vi "Receive TCP Message.vi"(3 "Error In":errorcluster, 4 "TCP Network Connection Refnum":refnum<k5>, 5 "Supervisor In":refnum<class "Supervisor.lvclass">) -> (0 "Error Out":errorcluster, 1 "TCP Network Connection Refnum Out":refnum<k5>, 2 "Supervisor Out":refnum<class "Supervisor.lvclass">)   [LabVIEW 2014, in "Supervisor.lvclass"]
uses:
  Supervisor.lvclass
  Supervisor.lvclass/Supervisor.ctl
panel:
  out "Numeric":i32
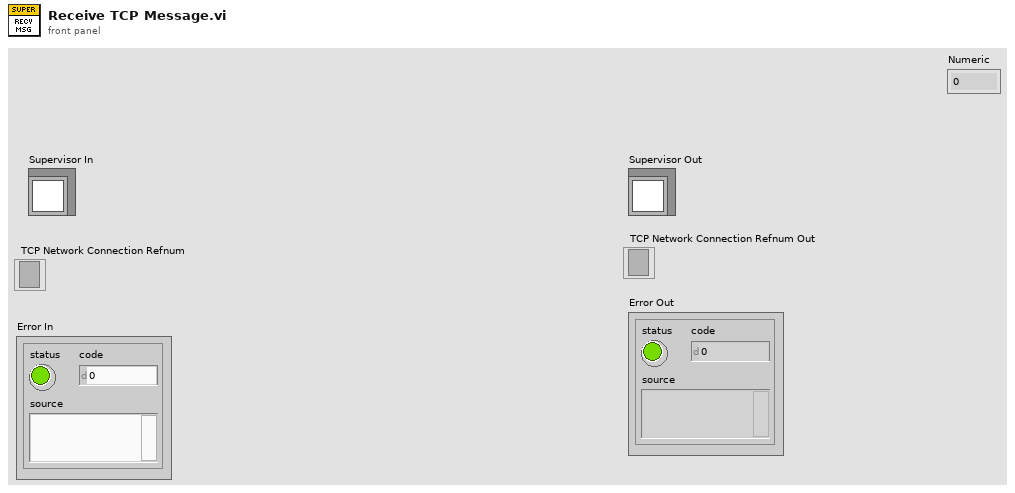
[diagram p1: front panel]
types:
  T1 = cluster{"javp":dbl[], " javr":dbl[], "Break":bool, "arrived":bool, "arrived yaw":bool}
  T2 = typedef "nicrio_cRIO-9871_BaudRateEnum.ctl" = enum16{"75 bps", "110 bps", "134 bps", "150 bps", "300 bps", "600 bps", "1200 bps", "1800 bps", "2400 bps", "4800 bps", "7200 bps", "9600 bps", "14.4 kbps", "19.2 kbps", "28.8 kbps", "38.4 kbps", "57.6 kbps", "115.2 kbps", "230.4 kbps", "460.8 kbps", "921.6 kbps"}
  T3 = typedef "nicrio_cRIO-9871_DataBitsEnum.ctl" = enum8{"5", "6", "7", "8"}
  T4 = typedef "nicrio_cRIO-9871_ParityEnum.ctl" = enum8{"None", "Odd", "Even", "Mark", "Space"}
  T5 = typedef "nicrio_cRIO-9871_StopBitsEnum.ctl" = enum8{"1", "1.5", "2"}
  T6 = typedef "nicrio_cRIO-9871_FlowControlEnum.ctl" = enum8{"None", "Software (XON / XOFF)", "Hardware (RTS / CTS)"}
  T7 = cluster{"Baud Rate":T2, "Data Bits":T3, "Parity":T4, "Stop Bits":T5, "Flow Control":T6}[]
  T8 = cluster{"Baud Rate":T2, "Data Bits":T3, "Parity":T4, "Stop Bits":T5, "Flow Control":T6}
  T9 = typedef "NI_Matrix.lvlib/RealMatrix.ctl" = dbl[][]
  T10 = cluster{"Performance Behavior":cluster{"% Velocity max lin to exp":dbl, "% Velocity zero lin to exp":dbl, "% Total dist at max velocity":dbl, "Max angular velocity":dbl, "Time to max linear velocity":dbl, "Min dist at max velocity":dbl, "Max linear velocity":dbl, "Time to max angular velocity":dbl}, "Table of WP":dbl[][], "Tracking Options":cluster{"Superior Bound":dbl, "Inferior Bound":dbl, "Duration No operation period between motions":dbl, "Tolerance of initial angle":dbl, "Distance to activation waiting function":dbl, "Distance to deactivation waiting function":dbl, "(2) Fixed Heading":dbl, "(3) PoI N":dbl, "(3) PoI E":dbl}, "Start":bool, "Use Position":bool, "Heading Mode":u16, "Pause":bool, "Abort":bool}
  T11 = cluster{"R":T9, "Q":T9, "Update R":bool, "Update Q":bool, "Name":string}
  T12 = cluster{"KP":T9, "KD":T9, "KI":T9, "KA":T9, "Update KP":bool, "Update KD":bool, "Update KI":bool, "Update KA":bool, "Name":string}
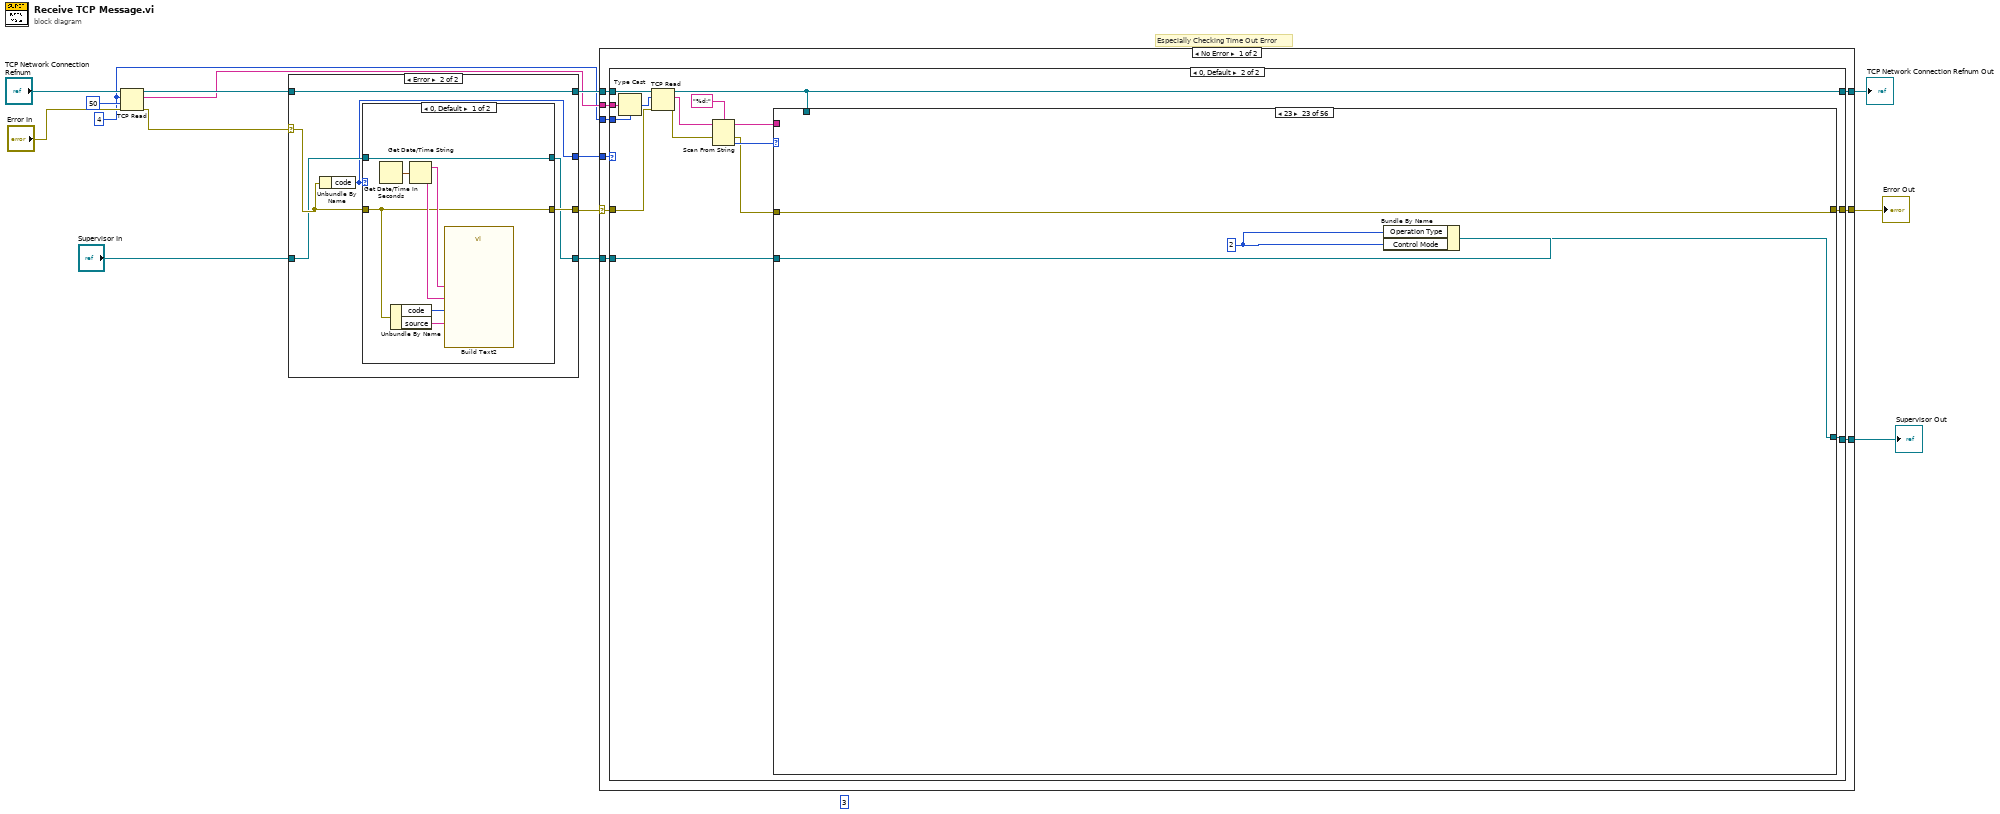
[diagram p0: block diagram]
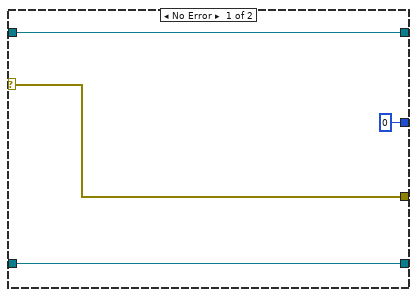
[diagram p2: hidden frame]
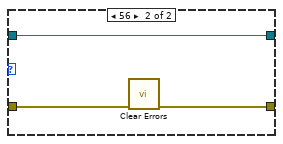
[diagram p3: hidden frame]
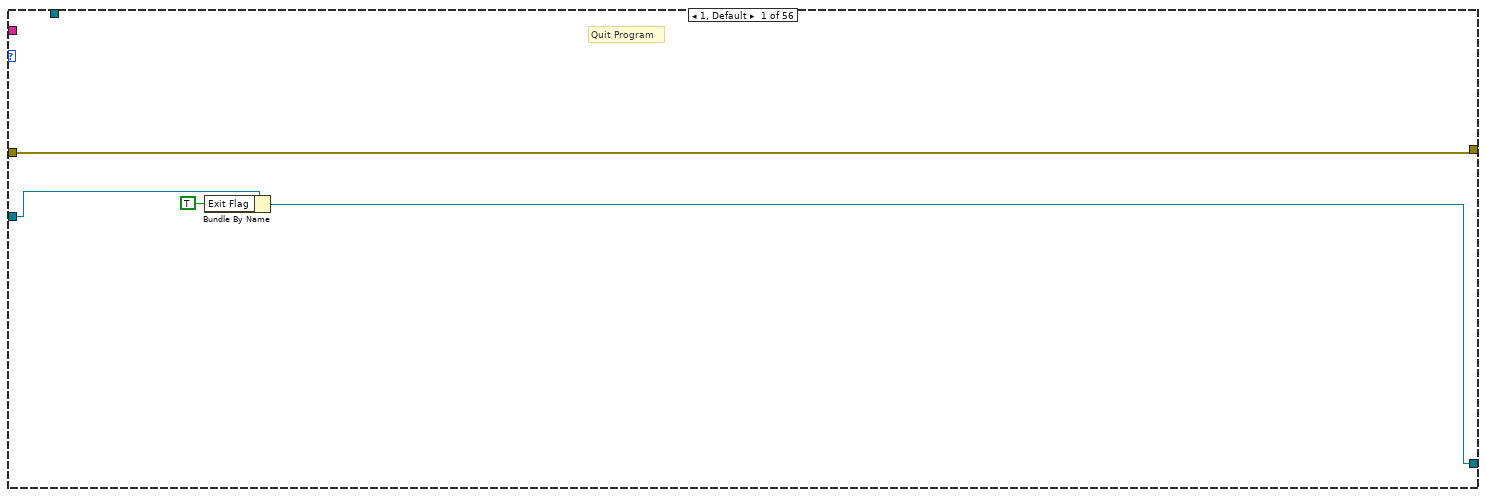
[diagram p5: hidden frame]
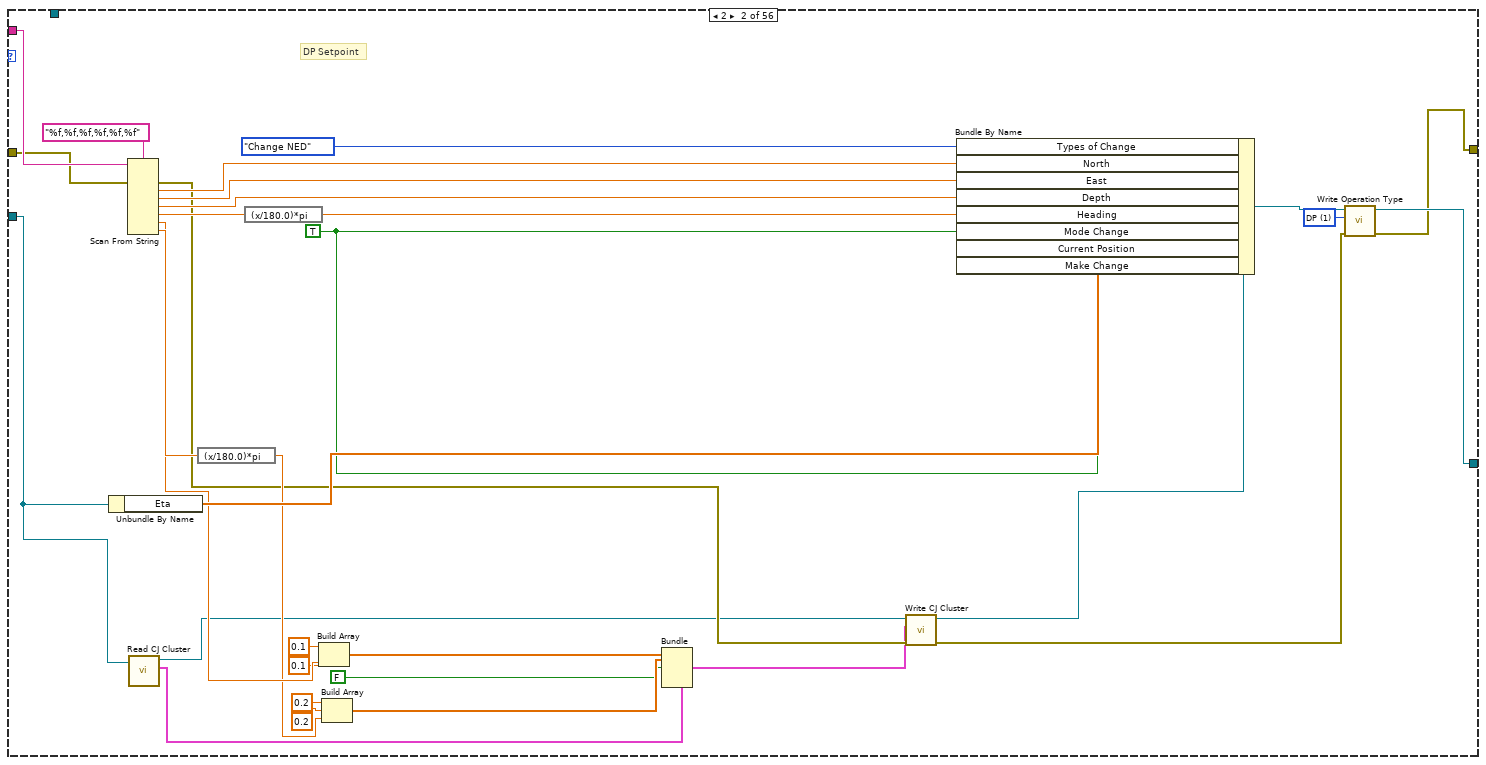
[diagram p6: hidden frame]
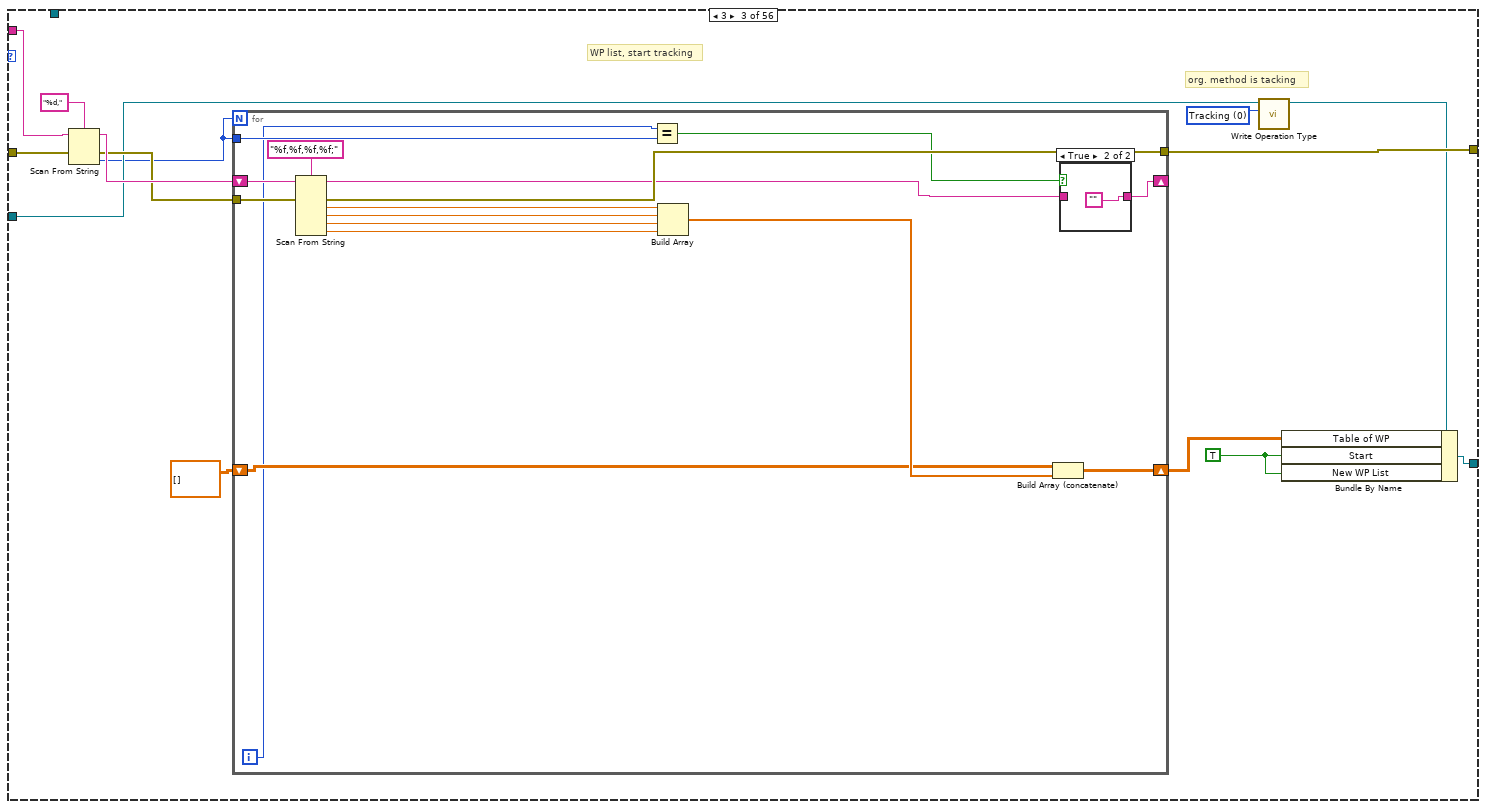
[diagram p7: hidden frame]
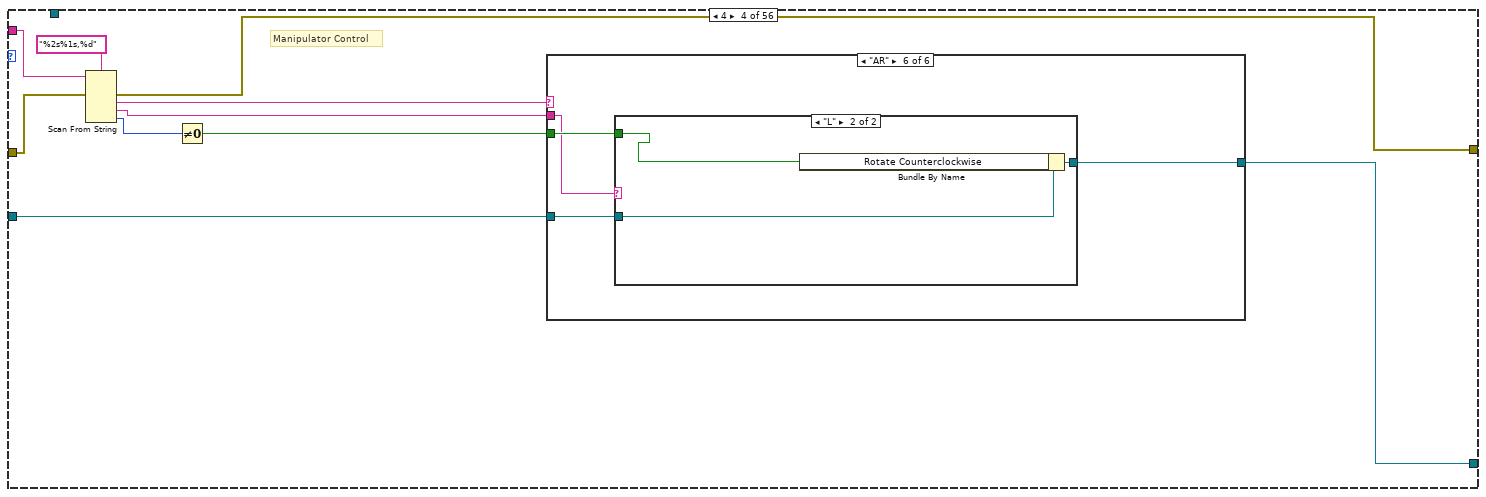
[diagram p9: hidden frame]
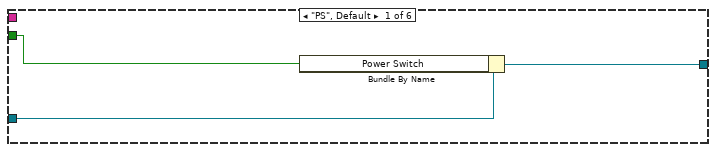
[diagram p10: hidden frame]
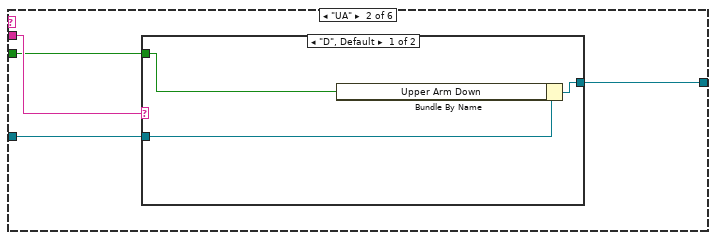
[diagram p11: hidden frame]
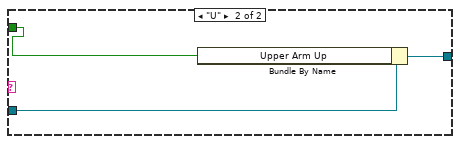
[diagram p12: hidden frame]
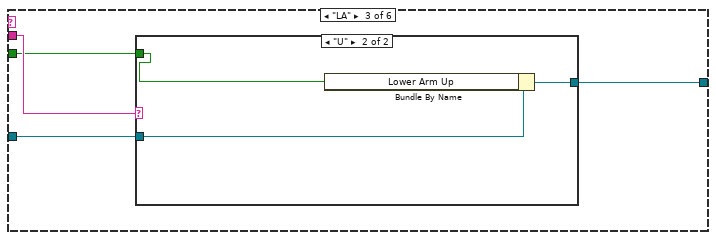
[diagram p13: hidden frame]
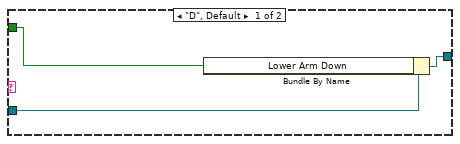
[diagram p14: hidden frame]
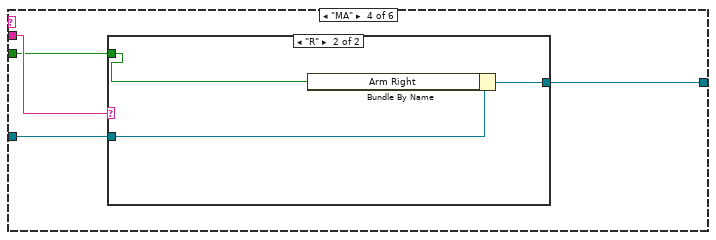
[diagram p15: hidden frame]
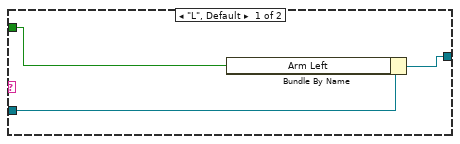
[diagram p16: hidden frame]
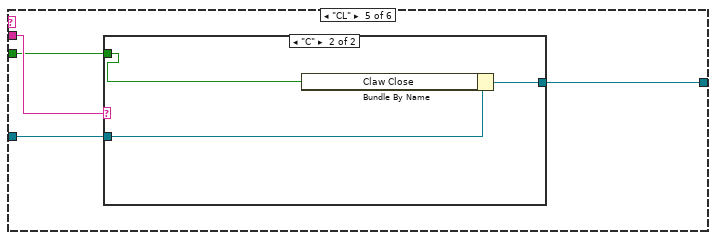
[diagram p17: hidden frame]
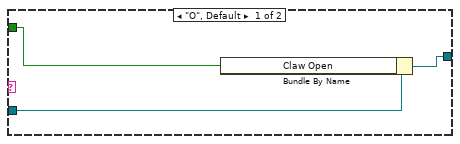
[diagram p18: hidden frame]
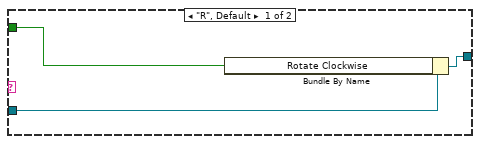
[diagram p19: hidden frame]
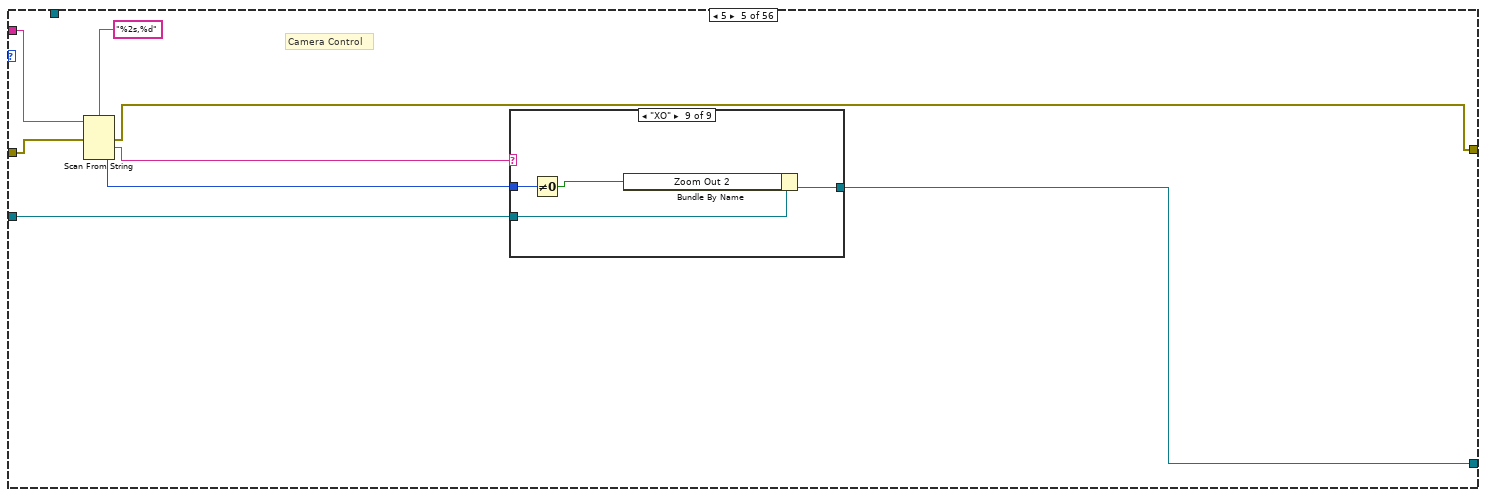
[diagram p20: hidden frame]
diagram:
  (unwired) 3
  w2 = 4
  # "Especially Checking Time Out Error"
  n1 = TCP Read(connection ID="TCP Network Connection Refnum", bytes to read=w2, error in (no error)="Error In", 9:50 ("timeout ms (25000)")) -> (connection ID out=w6:refnum<k5>, data out=w4:string, error out=w5:errorcluster)  [unwired: 1 in]
  n2 = case shown="Error" w5 {
    selector: w5 -> [w17 w24]
    tunnel: w6 -> [w19 w25]
    tunnel: [w19 w25] -> w9
    tunnel: [w18 w21] -> w8
    tunnel: [w17 w23] -> w3
    tunnel: "Supervisor In" -> [w18 w22]
    tunnel: [0 ("code") w20] -> w1
    frame No Error {
    }
    frame Error {
      n3 = Unbundle By Name(w24) -> ("code"=w20:i32)
      n4 = case shown="0, Default" w20 {
        tunnel: w24 -> [w29 w35]
        tunnel: [w29 w34] -> w23
        tunnel: w22 -> [w26 w33]
        tunnel: [w26 w33] -> w21
        frame 0, Default {
          n5 = Get Date/Time In Seconds() -> (seconds since 1Jan1904=w32:timestamp)
          n6 = Unbundle By Name(w29) -> ("code"=w28:i32, "source"=w27:string)
          n7 = Get Date/Time String(seconds (now)=w32) -> (date string=w31:string, time string=w30:string)  [unwired: 2 in]
          n8 = call "Build Text2"("Msg"=w27, "Date"=w31, "Time"=w30, "Code"=w28) -> ()  [unwired: 10 in, 2 out]
        }
        frame 56 {
          n9 = call <vilib>:"Clear Errors.vi"("error in (no error)"=w35) -> ("error out"=w34:errorcluster)  [unwired: 5 in, 1 out]
        }
      }
    }
  }
  n10 = case shown="No Error" w3 {
    selector: w3 -> [w38 w1206]
    tunnel: w9 -> [w44 w1210]
    tunnel: w4 -> [w43 _]
    tunnel: w2 -> [w42 _]
    tunnel: [w41 w1210] -> w14
    tunnel: [w40 w1207] -> w13
    tunnel: [w39 w1205] -> w11
    tunnel: w8 -> [w37 w1208]
    tunnel: w1 -> [w36 _]
    frame No Error {
      n11 = case shown="0, Default" w36 {
        tunnel: w44 -> [w47 w62]
        tunnel: w43 -> [_ w61]
        tunnel: w42 -> [_ w60]
        tunnel: [w47 w48] -> w41
        tunnel: [w45 w54] -> w40
        tunnel: [w46 w51] -> w39
        tunnel: w38 -> [w46 w50]
        tunnel: w37 -> [w45 w49]
        frame 56 {
        }
        frame 0, Default {
          n12 = Type Cast(type=w60, x=w61) -> (*(type *) &x=w59:i32)
          n13 = TCP Read(connection ID=w62, bytes to read=w59, error in (no error)=w50) -> (connection ID out=w48:refnum<k5>, data out=w58:string, error out=w53:errorcluster)  [unwired: 2 in]
          n14 = Scan From String(format string="%d:", input string=w58, error in=w53) -> (remaining string=w55:string, error out=w52:errorcluster, output 1=w56:i32)  [unwired: 2 in, 1 out]
          n15 = case shown="23" w56 {
            selector: w56 -> [_ _ _ _ _ _ w297 _ _ _ _ _ _ _ _ _ _ _ _ _ _ _ _ _ _ _ _ _ _ _ _ _ _ _ _ _ _ _ _ _ _ _ _ _ _ _ _ _ _ _ _ _ _ _ _ _]
            tunnel: w55 -> [_ w97 w111 w140 w199 w244 _ w307 w366 w420 w446 w466 w473 w483 w495 _ _ _ w529 w756 w764 w769 _ w782 w790 w795 w805 w809 w817 w827 w835 w843 w851 w859 w872 w911 w919 _ w943 w967 w976 w997 w1008 w1016 w1033 w1039 w1048 w1056 _ _ w1157 w1164 w1176 w1186 w1191 w1202]
            tunnel: w49 -> [w66 w68 w103 w134 w201 w240 w296 w302 w364 w418 w447 w463 w475 w480 w491 w509 w512 w516 w528 w753 w761 w768 w776 w779 w792 w797 w804 w813 w821 w829 w837 w845 w853 w861 w867 w908 w914 w923 w946 w968 w974 w985 w1007 w1015 w1031 w1037 w1043 w1054 w1086 w1122 w1161 w1169 w1174 w1183 w1190 w1199]
            tunnel: [w64 w88 w107 w133 w196 w239 w296 w301 w363 w416 w439 w459 w469 w476 w487 w507 w511 w515 w527 w751 w759 w766 w774 w777 w791 w796 w803 w812 w820 w828 w836 w841 w852 w860 w865 w906 w912 w923 w940 w966 w973 w982 w1000 w1013 w1024 w1035 w1045 w1053 w1086 w1122 w1160 w1163 w1173 w1184 w1189 w1197] -> w54
            tunnel: w52 -> [w63 w90 w106 w132 w195 w238 w295 w300 w365 w415 w444 w461 w474 w484 w492 w506 w513 w517 w526 w750 w758 w770 w773 w781 w786 w794 w802 w811 w819 w826 w834 w844 w850 w858 w871 w905 w917 w922 w947 w969 w975 w996 w1009 w1017 w1032 w1038 w1047 w1052 w1088 w1149 w1156 w1168 w1177 w1185 w1192 w1203]
            tunnel: [w63 w74 w104 w131 w194 w237 w295 w298 w394 w414 w443 w458 w467 w479 w490 w506 w513 w517 w524 w749 w757 w765 w773 w780 w785 w793 w801 w810 w818 w825 w833 w842 w849 w857 w870 w904 w915 w921 w939 w965 w972 w981 w999 w1014 w1025 w1036 w1046 w1050 w1087 w1148 w1162 w1166 w1171 w1180 w1193 w1198] -> w51
            tunnel: w48 -> [_ _ _ _ _ _ _ _ _ _ _ _ _ _ _ _ _ _ _ _ _ _ _ _ _ _ _ _ _ _ _ _ _ _ _ _ _ w920 _ _ _ _ _ _ _ _ _ _ w1089 w1150 _ _ _ _ _ _]
            frame 1, Default {
              # "Quit Program"
              n16 = Bundle By Name(cluster=w66, "Exit Flag"=TRUE) -> (w64:refnum<class "Supervisor.lvclass">)
            }
            frame 2 {
              w87 = u16 1 items=["Tracking", "DP", "Joystick"] ("Operation Type")
              w91 = TRUE ("Guidance Cluster.Update Reference.Mode Change")
              # "DP Setpoint"
              n17 = Unbundle By Name(w68) -> ("Eta"=w92:dbl[])
              n18 = Scan From String(format string="%f,%f,%f,%f,%f,%f", input string=w97, error in=w90) -> (error out=w75:errorcluster, output 1=w96:dbl, output 2=w95:dbl, output 3=w94:dbl, output 4=w85:dbl, output 5=w83:dbl, output 6=w84:dbl)  [unwired: 7 in, 2 out]
              n19 = call-dynamic "Read CJ Cluster.vi"("Supervisor in"=w68) -> ("CJ Cluster"=w71:T1, "Supervisor out"=w67:refnum<class "Supervisor.lvclass">)  [unwired: 8 in, 1 out]
              n20 = expression code="(x/180.0)*pi" ("degrees to radians")(w84) -> (w78:dbl)
              n21 = expression code="(x/180.0)*pi" ("degrees to radians")(w85) -> (w86:dbl)
              n22 = Build Array(0.1 ("element"), 0.1 ("element"), w83) -> (w77:dbl[])
              n23 = Build Array(0.2 ("element"), 0.2 ("element"), w78) -> (w73:dbl[])
              n24 = Bundle(cluster=w71, "javp"=w77, "javr"=w73, "Break"=FALSE ("Guidance Cluster.Update Reference.Mode Change")) -> (w70:T1)  [unwired: 2 in]
              n25 = call-dynamic "Write CJ Cluster.vi"("error in (no error)"=w75, "CJ Cluster"=w70, "Supervisor in"=w67) -> ("error out"=w76:errorcluster, "Supervisor out"=w72:refnum<class "Supervisor.lvclass">)  [unwired: 7 in]
              n26 = Bundle By Name(cluster=w72, "Types of Change"=enum16{"Current NED", "Change NED"}."Change NED" ("Guidance Cluster.Types of Change"), "North"=w96, "East"=w95, "Depth"=w94, "Heading"=w86, "Mode Change"=w91, "Current Position"=w92, "Make Change"=w91) -> (w89:refnum<class "Supervisor.lvclass">)
              n27 = call-dynamic "Write Operation Type.vi"("error in (no error)"=w76, "Operation Type"=w87, "Supervisor in"=w89) -> ("error out"=w74:errorcluster, "Supervisor out"=w88:refnum<class "Supervisor.lvclass">)  [unwired: 7 in]
            }
            frame 3 {
              w100 = TRUE ("Tracking Cluster.Start")
              w101 = u16 0 items=["Tracking", "DP", "Joystick"] ("Operation Type")
              # "org. method is tacking"
              # "WP list, start tracking"
              n28 = Scan From String(format string="%d,", input string=w111, error in=w106) -> (remaining string=w110:string, error out=w105:errorcluster, output 1=w99:i32)  [unwired: 2 in, 1 out]
              n29 = for {
                N: w99 -> [_]
                shift-right: [w121] -> w108
                shift-left: dbl[][] [] -> [w120]
                tunnel: w105 -> [w119]
                tunnel: [w118] -> w104
                shift-right: [w116] -> _
                shift-left: w110 -> [w127]
                tunnel: w99 -> [w115]
                i -> [w113]
                n30 = Scan From String(format string="%f,%f,%f,%f;", input string=w127, error in=w119) -> (remaining string=w117:string, error out=w118:errorcluster, output 1=w123:dbl, output 2=w126:dbl, output 3=w125:dbl, output 4=w124:dbl)  [unwired: 5 in, 1 out]
                n31 = Equal?(x=w113, y=w115) -> (x = y?=w114:bool)
                n32 = Build Array(w123, w126, w125, w124) -> (w122:dbl[])
                n33 = Build Array (concatenate)(w120, w122) -> (w121:dbl[][])
                n34 = case shown="True" w114 {
                  tunnel: w117 -> [w129 _]
                  tunnel: [w129 ""] -> w116
                  frame False {
                  }
                  frame True {
                  }
                }
              }
              n35 = call-dynamic "Write Operation Type.vi"("Operation Type"=w101, "Supervisor in"=w103) -> ("Supervisor out"=w102:refnum<class "Supervisor.lvclass">)  [unwired: 8 in, 1 out]
              n36 = Bundle By Name(cluster=w102, "Table of WP"=w108, "Start"=w100, "New WP List"=w100) -> (w107:refnum<class "Supervisor.lvclass">)
            }
            frame 4 {
              # "Manipulator Control"
              n37 = Scan From String(format string="%2s%1s,%d", input string=w140, error in=w132) -> (error out=w131:errorcluster, output 1=w138:string, output 2=w135:string, output 3=w136:i32)  [unwired: 4 in, 2 out]
              n38 = Not Equal To 0?(x=w136) -> (x != 0?=w137:bool)
              n39 = case shown="\"AR\"" w138 {
                tunnel: w137 -> [w142 w145 w156 w165 w175 w186]
                tunnel: w135 -> [_ w147 w157 w166 w176 w185]
                tunnel: w134 -> [w143 w146 w155 w167 w177 w187]
                tunnel: [w141 w144 w154 w164 w174 w184] -> w133
                frame "PS", Default {
                  n40 = Bundle By Name(cluster=w143, "Power Switch"=w142) -> (w141:refnum<class "Supervisor.lvclass">)
                }
                frame "UA" {
                  n41 = case shown="\"D\", Default" w147 {
                    tunnel: w146 -> [w150 w153]
                    tunnel: w145 -> [w149 w152]
                    tunnel: [w148 w151] -> w144
                    frame "D", Default {
                      n42 = Bundle By Name(cluster=w150, "Upper Arm Down"=w149) -> (w148:refnum<class "Supervisor.lvclass">)
                    }
                    frame "U" {
                      n43 = Bundle By Name(cluster=w153, "Upper Arm Up"=w152) -> (w151:refnum<class "Supervisor.lvclass">)
                    }
                  }
                }
                frame "LA" {
                  n44 = case shown="\"U\"" w157 {
                    tunnel: w155 -> [w160 w163]
                    tunnel: w156 -> [w159 w162]
                    tunnel: [w158 w161] -> w154
                    frame "D", Default {
                      n45 = Bundle By Name(cluster=w160, "Lower Arm Down"=w159) -> (w158:refnum<class "Supervisor.lvclass">)
                    }
                    frame "U" {
                      n46 = Bundle By Name(cluster=w163, "Lower Arm Up"=w162) -> (w161:refnum<class "Supervisor.lvclass">)
                    }
                  }
                }
                frame "MA" {
                  n47 = case shown="\"R\"" w166 {
                    tunnel: w167 -> [w170 w173]
                    tunnel: w165 -> [w169 w172]
                    tunnel: [w168 w171] -> w164
                    frame "L", Default {
                      n48 = Bundle By Name(cluster=w170, "Arm Left"=w169) -> (w168:refnum<class "Supervisor.lvclass">)
                    }
                    frame "R" {
                      n49 = Bundle By Name(cluster=w173, "Arm Right"=w172) -> (w171:refnum<class "Supervisor.lvclass">)
                    }
                  }
                }
                frame "CL" {
                  n50 = case shown="\"C\"" w176 {
                    tunnel: w177 -> [w180 w183]
                    tunnel: w175 -> [w179 w182]
                    tunnel: [w178 w181] -> w174
                    frame "O", Default {
                      n51 = Bundle By Name(cluster=w180, "Claw Open"=w179) -> (w178:refnum<class "Supervisor.lvclass">)
                    }
                    frame "C" {
                      n52 = Bundle By Name(cluster=w183, "Claw Close"=w182) -> (w181:refnum<class "Supervisor.lvclass">)
                    }
                  }
                }
                frame "AR" {
                  n53 = case shown="\"L\"" w185 {
                    tunnel: w187 -> [w190 w193]
                    tunnel: w186 -> [w189 w192]
                    tunnel: [w188 w191] -> w184
                    frame "R", Default {
                      n54 = Bundle By Name(cluster=w190, "Rotate Clockwise"=w189) -> (w188:refnum<class "Supervisor.lvclass">)
                    }
                    frame "L" {
                      n55 = Bundle By Name(cluster=w193, "Rotate Counterclockwise"=w192) -> (w191:refnum<class "Supervisor.lvclass">)
                    }
                  }
                }
              }
            }
            frame 5 {
              # "Camera Control"
              n56 = Scan From String(format string="%2s,%d", input string=w199, error in=w195) -> (error out=w194:errorcluster, output 1=w198:string, output 2=w197:i32)  [unwired: 3 in, 2 out]
              n57 = case shown="\"XO\"" w198 {
                tunnel: w201 -> [w204 w208 w211 w216 w219 w224 w228 w231 w236]
                tunnel: w197 -> [w203 w207 w212 w215 w220 w222 w226 w232 w234]
                tunnel: [w202 w205 w209 w213 w217 w223 w227 w230 w235] -> w196
                frame "CN", Default {
                  n58 = Bundle By Name(cluster=w204, "Cam. No."=w203) -> (w202:refnum<class "Supervisor.lvclass">)
                }
                frame "CU" {
                  n59 = Not Equal To 0?(x=w207) -> (x != 0?=w206:bool)
                  n60 = Bundle By Name(cluster=w208, "Cam Up"=w206) -> (w205:refnum<class "Supervisor.lvclass">)
                }
                frame "CD" {
                  n61 = Not Equal To 0?(x=w212) -> (x != 0?=w210:bool)
                  n62 = Bundle By Name(cluster=w211, "Cam Down"=w210) -> (w209:refnum<class "Supervisor.lvclass">)
                }
                frame "CR" {
                  n63 = Not Equal To 0?(x=w215) -> (x != 0?=w214:bool)
                  n64 = Bundle By Name(cluster=w216, "Cam Right"=w214) -> (w213:refnum<class "Supervisor.lvclass">)
                }
                frame "CL" {
                  n65 = Not Equal To 0?(x=w220) -> (x != 0?=w218:bool)
                  n66 = Bundle By Name(cluster=w219, "Cam Left"=w218) -> (w217:refnum<class "Supervisor.lvclass">)
                }
                frame "ZI" {
                  n67 = Not Equal To 0?(x=w222) -> (x != 0?=w221:bool)
                  n68 = Bundle By Name(cluster=w224, "Zoom In"=w221) -> (w223:refnum<class "Supervisor.lvclass">)
                }
                frame "ZO" {
                  n69 = Not Equal To 0?(x=w226) -> (x != 0?=w225:bool)
                  n70 = Bundle By Name(cluster=w228, "Zoom Out"=w225) -> (w227:refnum<class "Supervisor.lvclass">)
                }
                frame "XI" {
                  n71 = Not Equal To 0?(x=w232) -> (x != 0?=w229:bool)
                  n72 = Bundle By Name(cluster=w231, "Zoom In 2"=w229) -> (w230:refnum<class "Supervisor.lvclass">)
                }
                frame "XO" {
                  n73 = Not Equal To 0?(x=w234) -> (x != 0?=w233:bool)
                  n74 = Bundle By Name(cluster=w236, "Zoom Out 2"=w233) -> (w235:refnum<class "Supervisor.lvclass">)
                }
              }
            }
            frame 6 {
              # "Light Control"
              n75 = Scan From String(format string="%2s,%d", input string=w244, error in=w238) -> (error out=w237:errorcluster, output 1=w242:string, output 2=w241:i32)  [unwired: 3 in, 2 out]
              n76 = case shown="\"I1\", \"I2\", \"I3\"" w242 {
                selector: w242 -> [w249 w265]
                tunnel: w241 -> [w247 w262]
                tunnel: w240 -> [w245 w267]
                tunnel: [w246 w266] -> w239
                frame "I1", "I2", "I3" {
                  n77 = Decimal String To Number(string=w249, offset=1) -> (number=w248:i32)  [unwired: 1 in, 1 out]
                  n78 = case shown="3" w248 {
                    tunnel: w245 -> [w253 w256 w259]
                    tunnel: w247 -> [w252 w255 w258]
                    tunnel: [w251 w254 w257] -> w246
                    frame 2 {
                      n79 = Bundle By Name(cluster=w253, "Light Intensity 2"=w252) -> (w251:refnum<class "Supervisor.lvclass">)
                    }
                    frame 3 {
                      n80 = Bundle By Name(cluster=w256, "Light Intensity 3"=w255) -> (w254:refnum<class "Supervisor.lvclass">)
                    }
                    frame 1, Default {
                      n81 = Bundle By Name(cluster=w259, "Light Intensity 1"=w258) -> (w257:refnum<class "Supervisor.lvclass">)
                    }
                  }
                }
                frame "H~", "L~", Default {
                  n82 = Not Equal To 0?(x=w262) -> (x != 0?=w261:bool)
                  n83 = String Subset(string=w265, length (rest)=1 ("length (rest)")) -> (substring=w268:string)  [unwired: 1 in]
                  n84 = Decimal String To Number(string=w265, offset=1) -> (number=w264:i32)  [unwired: 1 in, 1 out]
                  n85 = case shown="\"L\", Default" w268 {
                    tunnel: w261 -> [w272 w286]
                    tunnel: w267 -> [w271 w287]
                    tunnel: [w270 w285] -> w266
                    tunnel: w264 -> [w269 w288]
                    frame "L", Default {
                      n86 = case shown="4" w269 {
                        tunnel: w272 -> [w274 w277 w280 w283]
                        tunnel: w271 -> [w275 w278 w281 w284]
                        tunnel: [w273 w276 w279 w282] -> w270
                        frame 1, Default {
                          n87 = Bundle By Name(cluster=w275, "Light 1"=w274) -> (w273:refnum<class "Supervisor.lvclass">)
                        }
                        frame 2 {
                          n88 = Bundle By Name(cluster=w278, "Light 2"=w277) -> (w276:refnum<class "Supervisor.lvclass">)
                        }
                        frame 3 {
                          n89 = Bundle By Name(cluster=w281, "Light 3"=w280) -> (w279:refnum<class "Supervisor.lvclass">)
                        }
                        frame 4 {
                          n90 = Bundle By Name(cluster=w284, "Light 4"=w283) -> (w282:refnum<class "Supervisor.lvclass">)
                        }
                      }
                    }
                    frame "H" {
                      n91 = case shown="2" w288 {
                        tunnel: w287 -> [w291 w294]
                        tunnel: w286 -> [w290 w293]
                        tunnel: [w289 w292] -> w285
                        frame 1, Default {
                          n92 = Bundle By Name(cluster=w291, "HMI 1"=w290) -> (w289:refnum<class "Supervisor.lvclass">)
                        }
                        frame 2 {
                          n93 = Bundle By Name(cluster=w294, "HMI 2"=w293) -> (w292:refnum<class "Supervisor.lvclass">)
                        }
                      }
                    }
                  }
                }
              }
            }
            frame 7 {
              # "YOYSTICK MESSAGES?"
              "Numeric" <- w297
            }
            frame 8 {
              n94 = Scan From String(format string="%3s,%f", input string=w307, error in=w300) -> (remaining string=w303:string, error out=w299:errorcluster, output 1=w305:string, output 2=w304:dbl)  [unwired: 3 in, 1 out]
              n95 = case shown="\"AWF\"" w305 {
                tunnel: w304 -> [w310 w315 w319 w323 w327 w331 w335 w339 w343 w347 w358]
                tunnel: w303 -> [_ _ _ _ _ _ _ _ _ _ w362]
                tunnel: w302 -> [w312 w316 w320 w324 w328 w332 w336 w340 w344 w348 w360]
                tunnel: [w311 w314 w318 w322 w326 w330 w334 w338 w342 w346 w359] -> w301
                tunnel: w299 -> [w308 w313 w317 w321 w325 w329 w333 w337 w341 w345 w350]
                tunnel: [w308 w313 w317 w321 w325 w329 w333 w337 w341 w345 w349] -> w298
                frame "HeM", Default {
                  n96 = To Long Integer(number=w310) -> (32bit integer=w309:i32)
                  n97 = Bundle By Name(cluster=w312, "Heading Mode"=w309) -> (w311:refnum<class "Supervisor.lvclass">)
                }
                frame "DFH" {
                  n98 = Bundle By Name(cluster=w316, "(2) Fixed Heading"=w315) -> (w314:refnum<class "Supervisor.lvclass">)
                }
                frame "PIN" {
                  n99 = Bundle By Name(cluster=w320, "(3) PoI N"=w319) -> (w318:refnum<class "Supervisor.lvclass">)
                }
                frame "PIE" {
                  n100 = Bundle By Name(cluster=w324, "(3) PoI E"=w323) -> (w322:refnum<class "Supervisor.lvclass">)
                }
                frame "SuB" {
                  n101 = Bundle By Name(cluster=w328, "Superior Bound"=w327) -> (w326:refnum<class "Supervisor.lvclass">)
                }
                frame "InB" {
                  n102 = Bundle By Name(cluster=w332, "Inferior Bound"=w331) -> (w330:refnum<class "Supervisor.lvclass">)
                }
                frame "NOP" {
                  n103 = Bundle By Name(cluster=w336, "Duration No operation period between motions"=w335) -> (w334:refnum<class "Supervisor.lvclass">)
                }
                frame "TIA" {
                  n104 = Bundle By Name(cluster=w340, "Tolerance of initial angle"=w339) -> (w338:refnum<class "Supervisor.lvclass">)
                }
                frame "AWF" {
                  n105 = Bundle By Name(cluster=w344, "Distance to activation waiting function"=w343) -> (w342:refnum<class "Supervisor.lvclass">)
                }
                frame "DWF" {
                  n106 = Bundle By Name(cluster=w348, "Distance to deactivation waiting function"=w347) -> (w346:refnum<class "Supervisor.lvclass">)
                }
                frame "UDB" {
                  n107 = Scan From String(format string="%f,%f,%f,%f,%f,%f,%f", input string=w362, error in=w350) -> (error out=w349:errorcluster, output 1=w357:dbl, output 2=w356:dbl, output 3=w355:dbl, output 4=w354:dbl, output 5=w353:dbl, output 6=w352:dbl, output 7=w351:dbl)  [unwired: 8 in, 2 out]
                  n108 = Bundle By Name(cluster=w360, "% Velocity max lin to exp"=w354, "% Velocity zero lin to exp"=w353, "% Total dist at max velocity"=w355, "Max angular velocity"=w352, "Time to max linear velocity"=w357, "Min dist at max velocity"=w356, "Max linear velocity"=w358, "Time to max angular velocity"=w351) -> (w359:refnum<class "Supervisor.lvclass">)
                }
              }
            }
            frame 9 {
              w385 = u16 1 items=["Tracking", "DP", "Joystick"] ("Operation Type")
              w387 = TRUE ("Guidance Cluster.Update Reference.Mode Change")
              n109 = disable-structure shown="Disabled" {
                disable-tunnel: [w399 _] -> _
                disable-tunnel: [w398 _] -> w394
                disable-tunnel: w366 -> [w397 _]
                disable-tunnel: w365 -> [w396 _]
                disable-tunnel: w364 -> [w395 _]
                frame Disabled {
                  n110 = Scan From String(format string="%1s,%d", input string=w397, error in=w396) -> (error out=w398:errorcluster, output 1=w402:string, output 2=w401:i32)  [unwired: 3 in, 2 out]
                  n111 = Not Equal To 0?(x=w401) -> (x != 0?=w400:bool)
                  n112 = case shown="\"A\", Default" w402 {
                    tunnel: w400 -> [w405 w410]
                    tunnel: w395 -> [w406 w411]
                    tunnel: [w404 w407] -> w399
                    frame "A", Default {
                      n113 = Bundle By Name(cluster=w406, "Abort"=w405) -> (w404:refnum<class "Supervisor.lvclass">)
                    }
                    frame "P" {
                      w409 = u16 0 items=["Tracking", "DP", "Joystick"] ("Operation Type")
                      n114 = Bundle By Name(cluster=w411, "Pause"=w410) -> (w408:refnum<class "Supervisor.lvclass">)
                      n115 = call-dynamic "Write Operation Type.vi"("Operation Type"=w409, "Supervisor in"=w408) -> ("Supervisor out"=w407:refnum<class "Supervisor.lvclass">)  [unwired: 8 in, 1 out]
                    }
                  }
                }
                frame Enabled {
                }
              }
              n116 = Unbundle By Name(w364) -> ("Eta"=w388:dbl[])
              n117 = Scan From String(format string="%f,%f,%f,%f,%f,%f", input string=w366, error in=w365) -> (error out=w373:errorcluster, output 1=w392:dbl, output 2=w391:dbl, output 3=w390:dbl, output 4=w383:dbl, output 5=w381:dbl, output 6=w382:dbl)  [unwired: 7 in, 2 out]
              n118 = call-dynamic "Read CJ Cluster.vi"("Supervisor in"=w364) -> ("CJ Cluster"=w370:T1, "Supervisor out"=w367:refnum<class "Supervisor.lvclass">)  [unwired: 8 in, 1 out]
              n119 = expression code="(x/180.0)*pi" ("degrees to radians")(w382) -> (w376:dbl)
              n120 = expression code="(x/180.0)*pi" ("degrees to radians")(w383) -> (w384:dbl)
              n121 = Build Array(0.1 ("element"), 0.1 ("element"), w381) -> (w375:dbl[])
              n122 = Build Array(0.2 ("element"), 0.2 ("element"), w376) -> (w372:dbl[])
              n123 = Bundle(cluster=w370, "javp"=w375, "javr"=w372, "Break"=FALSE ("Guidance Cluster.Update Reference.Mode Change")) -> (w369:T1)  [unwired: 2 in]
              n124 = call-dynamic "Write CJ Cluster.vi"("error in (no error)"=w373, "CJ Cluster"=w369, "Supervisor in"=w367) -> ("error out"=w374:errorcluster, "Supervisor out"=w371:refnum<class "Supervisor.lvclass">)  [unwired: 7 in]
              n125 = Bundle By Name(cluster=w371, "Types of Change"=enum16{"Current NED", "Change NED"}."Change NED" ("Guidance Cluster.Types of Change"), "North"=w392, "East"=w391, "Depth"=w390, "Heading"=w384, "Mode Change"=w387, "Current Position"=w388, "Make Change"=w387) -> (w386:refnum<class "Supervisor.lvclass">)
              n126 = call-dynamic "Write Operation Type.vi"("error in (no error)"=w374, "Operation Type"=w385, "Supervisor in"=w386) -> ("Supervisor out"=w363:refnum<class "Supervisor.lvclass">)  [unwired: 7 in, 1 out]
            }
            frame 10 {
              # "Port Configuration Update"
              # "Number of Ports"
              n127 = Unbundle By Name(w418) -> ("Updated Port Configurations"=w419:T7)
              n128 = Index Array(array=w419) -> (element=w421:T8)  [unwired: 1 in]
              n129 = for {
                N: 8 -> [_]
                tunnel: w421 -> [w437]
                shift-right: [w435] -> _
                shift-left: w420 -> [w436]
                shift-right: [w424] -> w417
                shift-left: w419 -> [w428]
                tunnel: w415 -> [w423]
                tunnel: [w422] -> w414
                n130 = Scan From String(format string="%d,%d,%d,%d,%d,%d;", input string=w436, error in=w423) -> (remaining string=w435:string, error out=w422:errorcluster, output 1=w426:i32, output 2=w433:i32, output 3=w432:i32, output 4=w431:i32, output 5=w430:i32, output 6=w429:i32)  [unwired: 7 in, 1 out]
                n131 = Bundle By Name(cluster=w437, "Baud Rate"=w433, "Data Bits"=w432, "Parity"=w431, "Stop Bits"=w430, "Flow Control"=w429) -> (w427:T8)
                n132 = Decrement(x=w426) -> (x-1=w425:i32)
                n133 = Insert Into Array(array=w428, index=w425, new element=w427) -> (w424:T7)
              }
              n134 = Bundle By Name(cluster=w418, "Updated Port Configurations"=w417, "Update Ports"=TRUE) -> (w416:refnum<class "Supervisor.lvclass">)
            }
            frame 11 {
              # "This will signal the system to update the origion coordinates."
              # "Set Origin command"
              n135 = Scan From String(format string="%d,", input string=w446, error in=w444) -> (remaining string=w440:string, error out=w443:errorcluster, output 1=w438:i32)  [unwired: 2 in, 1 out]
              n136 = Bundle By Name(cluster=w447, "Set Origin"=TRUE ("Guidance Cluster.Set Origin")) -> (w441:refnum<class "Supervisor.lvclass">)
              n137 = case shown="1" w438 {
                selector: w438 -> [w450 w451]
                tunnel: w441 -> [w449 w455]
                tunnel: w440 -> [_ w457]
                tunnel: [w448 w452] -> w439
                frame 0, 2, Default {
                  n138 = Bundle By Name(cluster=w449, "Coordinate System"=w450) -> (w448:refnum<class "Supervisor.lvclass">)
                }
                frame 1 {
                  n139 = Scan From String(format string="%f,%f", input string=w457) -> (output 1=w454:dbl, output 2=w453:dbl)  [unwired: 4 in, 3 out]
                  n140 = Bundle By Name(cluster=w455, "North"=w454, "East"=w453, "Coordinate System"=w451) -> (w452:refnum<class "Supervisor.lvclass">)
                }
              }
            }
            frame 12 {
              n141 = Scan From String(format string="%d", input string=w466, error in=w461) -> (error out=w460:errorcluster, output 1=w464:i32)  [unwired: 2 in, 2 out]
              n142 = Not Equal To 0?(x=w464) -> (x != 0?=w462:bool)
              n143 = call-dynamic "Write Use Estimated Values.vi"("error in (no error)"=w460, "Estimated Values"=w462, "Supervisor in"=w463) -> ("error out"=w458:errorcluster, "Supervisor out"=w459:refnum<class "Supervisor.lvclass">)  [unwired: 7 in]
            }
            frame 13 {
              n144 = Scan From String(format string="%d", input string=w473, error in=w474) -> (error out=w468:errorcluster, output 1=w471:i32)  [unwired: 2 in, 2 out]
              n145 = To Unsigned Word Integer(number=w471) -> (unsigned 16bit integer=w470:u16)
              n146 = call-dynamic "Write Frame Mode.vi"("error in (no error)"=w468, "Frame Mode"=w470, "Supervisor in"=w475) -> ("error out"=w467:errorcluster, "Supervisor out"=w469:refnum<class "Supervisor.lvclass">)  [unwired: 7 in]
            }
            frame 14 {
              n147 = Scan From String(format string="%d", input string=w483, error in=w484) -> (error out=w478:errorcluster, output 1=w481:i32)  [unwired: 2 in, 2 out]
              n148 = To Unsigned Word Integer(number=w481) -> (unsigned 16bit integer=w477:u16)
              n149 = call-dynamic "Write Control Mode.vi"("error in (no error)"=w478, "Control Mode"=w477, "Supervisor in"=w480) -> ("error out"=w479:errorcluster, "Supervisor out"=w476:refnum<class "Supervisor.lvclass">)  [unwired: 7 in]
            }
            frame 15 {
              n150 = Scan From String(format string="%d,%d,", input string=w495, error in=w492) -> (remaining string=w488:string, error out=w490:errorcluster, output 1=w493:i32, output 2=w486:i32)  [unwired: 3 in, 1 out]
              n151 = Not Equal To 0?(x=w493) -> (x != 0?=w485:bool)
              n152 = Bundle By Name(cluster=w491, "Reset ROV"=w485, "Reset Controller"=w485, "Reset Observer"=w485, "Set Origin"=w485, "Control System Active"=w485) -> (w489:refnum<class "Supervisor.lvclass">)
              n153 = case shown="1" w486 {
                selector: w486 -> [w497 w499]
                tunnel: w489 -> [w498 w505]
                tunnel: w488 -> [_ w504]
                tunnel: [w496 w500] -> w487
                frame 0, 2, Default {
                  n154 = Bundle By Name(cluster=w498, "Coordinate System"=w497) -> (w496:refnum<class "Supervisor.lvclass">)
                }
                frame 1 {
                  n155 = Scan From String(format string="%f,%f", input string=w504) -> (output 1=w502:dbl, output 2=w501:dbl)  [unwired: 4 in, 3 out]
                  n156 = Bundle By Name(cluster=w505, "North"=w502, "East"=w501, "Coordinate System"=w499) -> (w500:refnum<class "Supervisor.lvclass">)
                }
              }
            }
            frame 16 {
              # "Reset Observer"
              n157 = Bundle By Name(cluster=w509, "Reset Observer"=TRUE) -> (w507:refnum<class "Supervisor.lvclass">)
            }
            frame 17 {
              # "Reset Controller"
              n158 = Bundle By Name(cluster=w512, "Reset Controller"=TRUE) -> (w511:refnum<class "Supervisor.lvclass">)
            }
            frame 18 {
              w514 = TRUE ("Reset ROV")
              # "Reset ROV"
              n159 = Bundle By Name(cluster=w516, "Reset ROV"=w514, "Reset Controller"=w514) -> (w515:refnum<class "Supervisor.lvclass">)
            }
            frame 19 {
              n160 = Scan From String(format string="%3s", input string=w529, error in=w526) -> (remaining string=w523:string, error out=w525:errorcluster, output 1=w530:string)  [unwired: 2 in, 1 out]
              n161 = Search/Split String(string=w523, search string/char (-)="-") -> (substring before match=w522:string, match + rest of string=w520:string)  [unwired: 1 in, 1 out]
              n162 = String Subset(string=w520, offset (0)=1) -> (substring=w518:string)  [unwired: 1 in]
              n163 = case shown="\"KFR\", Default" w530 {
                tunnel: w522 -> [w537 w580 w628 w673 w725]
                tunnel: w528 -> [w536 w579 w627 w672 w724]
                tunnel: [w535 w578 w626 w671 w723] -> w527
                tunnel: w525 -> [w534 w577 w625 w670 w722]
                tunnel: [w533 w576 w624 w669 w721] -> w524
                tunnel: w518 -> [w532 w575 w623 w668 _]
                frame "KFR", Default {
                  n164 = while {
                    shift-right: [w546] -> _
                    shift-left: w537 -> [w558]
                    shift-right: [w543] -> w535
                    shift-left: w536 -> [w540]
                    shift-right: [w541] -> w533
                    shift-left: w534 -> [w542]
                    tunnel: w532 -> [w538]
                    stop <- w554 continue-if-true
                    n165 = Search/Split String(string=w558, search string/char (-)=",") -> (substring before match=w552:string, match + rest of string=w547:string)  [unwired: 1 in, 1 out]
                    n166 = Scan From String(format string="%1s:%1s", input string=w552, error in=w542) -> (remaining string=w551:string, error out=w541:errorcluster, output 1=w549:string, output 2=w545:string)  [unwired: 3 in, 1 out]
                    n167 = case shown="\"Q\"" w545 {
                      tunnel: [12 ("Martix Dimension") 12 ("Martix Dimension")] -> w544
                      frame "R", Default {
                      }
                      frame "Q" {
                      }
                    }
                    n168 = Replace Substring(2:1 ("length (len. of substring)"), 5:w547) -> (1:w546:string)  [unwired: 2 in, 1 out]
                    n169 = case shown="\"N\", Default" w549 {
                      tunnel: w551 -> [w563 w566]
                      tunnel: [w562 w565] -> w550
                      tunnel: w544 -> [w561 w564]
                      frame "N", Default {
                        n170 = call "String to Matrix (Norm).vi"("Martix Dimension"=w561, "String"=w563) -> ("Output Matrix"=w562:T9)
                      }
                      frame "D" {
                        n171 = call "String to Matrix (Diag).vi"("Martix Dimension"=w564, "String Input"=w566) -> ("Matrix Out"=w565:T9)
                      }
                    }
                    n172 = Bundle By Name(cluster=w540, "Name"=w538) -> (w539:refnum<class "Supervisor.lvclass">)
                    n173 = case shown="\"R\", Default" w545 {
                      tunnel: w550 -> [w569 w573]
                      tunnel: w539 -> [w570 w574]
                      tunnel: [w567 w571] -> w543
                      frame "R", Default {
                        n174 = Bundle By Name(cluster=w570, "R"=w569, "Update R"=TRUE ("Kalman Filter Observer Tuning.Update R")) -> (w567:refnum<class "Supervisor.lvclass">)
                      }
                      frame "Q" {
                        n175 = Bundle By Name(cluster=w574, "Q"=w573, "Update Q"=TRUE ("Kalman Filter Observer Tuning.Update Q")) -> (w571:refnum<class "Supervisor.lvclass">)
                      }
                    }
                    n176 = String Length(string=w546) -> (length=w556:i32)
                    n177 = Greater?(x=w556, y=1) -> (0:w554:bool)
                  }
                }
                frame "NLP" {
                  n178 = while {
                    shift-right: [w587] -> _
                    shift-left: w580 -> [w600]
                    shift-right: [w586] -> w578
                    shift-left: w579 -> [w583]
                    shift-right: [w584] -> w576
                    shift-left: w577 -> [w585]
                    tunnel: w575 -> [w582]
                    stop <- w596 continue-if-true
                    n179 = Search/Split String(string=w600, search string/char (-)=",") -> (substring before match=w594:string, match + rest of string=w588:string)  [unwired: 1 in, 1 out]
                    n180 = Bundle By Name(cluster=w583, "Name"=w582) -> (w581:refnum<class "Supervisor.lvclass">)
                    n181 = Scan From String(format string="%1s:%1s", input string=w594, error in=w585) -> (remaining string=w593:string, error out=w584:errorcluster, output 1=w590:string, output 2=w591:string)  [unwired: 3 in, 1 out]
                    n182 = Replace Substring(2:1 ("length (len. of substring)"), 5:w588) -> (1:w587:string)  [unwired: 2 in, 1 out]
                    n183 = case shown="\"N\", Default" w590 {
                      tunnel: w593 -> [w603 w606]
                      tunnel: [w601 w604] -> w592
                      frame "N", Default {
                        n184 = call "String to Matrix (Norm).vi"("Martix Dimension"=6, "String"=w603) -> ("Output Matrix"=w601:T9)
                      }
                      frame "D" {
                        n185 = call "String to Matrix (Diag).vi"("Martix Dimension"=6, "String Input"=w606) -> ("Matrix Out"=w604:T9)
                      }
                    }
                    n186 = case shown="\"A\"" w591 {
                      tunnel: w592 -> [w609 w613 w617 w621]
                      tunnel: w581 -> [w610 w614 w618 w622]
                      tunnel: [w607 w611 w616 w619] -> w586
                      frame "P", Default {
                        n187 = Bundle By Name(cluster=w610, "KP"=w609, "Update KP"=TRUE) -> (w607:refnum<class "Supervisor.lvclass">)
                      }
                      frame "D" {
                        n188 = Bundle By Name(cluster=w614, "KD"=w613, "Update KD"=TRUE ("Non Linear PID Tuning.Update KD")) -> (w611:refnum<class "Supervisor.lvclass">)
                      }
                      frame "I" {
                        n189 = Bundle By Name(cluster=w618, "KI"=w617, "Update KI"=TRUE ("Non Linear PID Tuning.Update KI")) -> (w616:refnum<class "Supervisor.lvclass">)
                      }
                      frame "A" {
                        n190 = Bundle By Name(cluster=w622, "KA"=w621, "Update KA"=TRUE ("Non Linear PID Tuning.Update KA")) -> (w619:refnum<class "Supervisor.lvclass">)
                      }
                    }
                    n191 = String Length(string=w587) -> (length=w598:i32)
                    n192 = Greater?(x=w598, y=1) -> (0:w596:bool)
                  }
                }
                frame "LPI " {
                  n193 = while {
                    shift-right: [w636] -> _
                    shift-left: w628 -> [w649]
                    shift-right: [w632] -> w626
                    shift-left: w627 -> [w630]
                    shift-right: [w634] -> w624
                    shift-left: w625 -> [w635]
                    tunnel: w623 -> [w631]
                    stop <- w645 continue-if-true
                    n194 = Search/Split String(string=w649, search string/char (-)=",") -> (substring before match=w643:string, match + rest of string=w637:string)  [unwired: 1 in, 1 out]
                    n195 = Scan From String(format string="%1s:%1s", input string=w643, error in=w635) -> (remaining string=w642:string, error out=w634:errorcluster, output 1=w639:string, output 2=w640:string)  [unwired: 3 in, 1 out]
                    n196 = Replace Substring(2:1 ("length (len. of substring)"), 5:w637) -> (1:w636:string)  [unwired: 2 in, 1 out]
                    n197 = Bundle By Name(cluster=w630, "Name"=w631) -> (w629:refnum<class "Supervisor.lvclass">)
                    n198 = case shown="\"N\", Default" w639 {
                      tunnel: w642 -> [w652 w655]
                      tunnel: [w650 w653] -> w641
                      frame "N", Default {
                        n199 = call "String to Matrix (Norm).vi"("Martix Dimension"=6, "String"=w652) -> ("Output Matrix"=w650:T9)
                      }
                      frame "D" {
                        n200 = call "String to Matrix (Diag).vi"("Martix Dimension"=6, "String Input"=w655) -> ("Matrix Out"=w653:T9)
                      }
                    }
                    n201 = case shown="\"I\"" w640 {
                      tunnel: w641 -> [w658 w661 w666]
                      tunnel: w629 -> [w659 w663 w667]
                      tunnel: TRUE -> [w657 w662 w665]
                      tunnel: [w656 w660 w664] -> w632
                      frame "P", Default {
                        n202 = Bundle By Name(cluster=w659, "Update KP"=w657, "KP"=w658) -> (w656:refnum<class "Supervisor.lvclass">)
                      }
                      frame "D" {
                        n203 = Bundle By Name(cluster=w663, "Update KD"=w662, "KD"=w661) -> (w660:refnum<class "Supervisor.lvclass">)
                      }
                      frame "I" {
                        n204 = Bundle By Name(cluster=w667, "Update KI"=w665, "KI"=w666) -> (w664:refnum<class "Supervisor.lvclass">)
                      }
                    }
                    n205 = String Length(string=w636) -> (length=w647:i32)
                    n206 = Greater?(x=w647, y=1) -> (0:w645:bool)
                  }
                }
                frame "LQR" {
                  n207 = while {
                    shift-right: [w683] -> _
                    shift-left: w673 -> [w695]
                    shift-right: [w677] -> w671
                    shift-left: w672 -> [w676]
                    shift-right: [w679] -> w669
                    shift-left: w670 -> [w680]
                    tunnel: w668 -> [w674]
                    stop <- w691 continue-if-true
                    n208 = Search/Split String(string=w695, search string/char (-)=",") -> (substring before match=w689:string, match + rest of string=w684:string)  [unwired: 1 in, 1 out]
                    n209 = Scan From String(format string="%1s:%1s", input string=w689, error in=w680) -> (remaining string=w688:string, error out=w679:errorcluster, output 1=w686:string, output 2=w682:string)  [unwired: 3 in, 1 out]
                    n210 = case shown="\"A\", \"I\"" w682 {
                      tunnel: [6 ("Martix Dimension") 12 ("Martix Dimension") 6 ("Martix Dimension")] -> w681
                      frame "R", Default {
                      }
                      frame "Q" {
                      }
                      frame "A", "I" {
                      }
                    }
                    n211 = Replace Substring(2:1 ("length (len. of substring)"), 5:w684) -> (1:w683:string)  [unwired: 2 in, 1 out]
                    n212 = case shown="\"N\", Default" w686 {
                      tunnel: w688 -> [w701 w704]
                      tunnel: [w700 w702] -> w687
                      tunnel: w681 -> [w699 _]
                      frame "N", Default {
                        n213 = call "String to Matrix (Norm).vi"("Martix Dimension"=w699, "String"=w701) -> ("Output Matrix"=w700:T9)
                      }
                      frame "D" {
                        n214 = call "String to Matrix (Diag).vi"("Martix Dimension"=6, "String Input"=w704) -> ("Matrix Out"=w702:T9)
                      }
                    }
                    n215 = Bundle By Name(cluster=w676, "Name"=w674) -> (w675:refnum<class "Supervisor.lvclass">)
                    n216 = case shown="\"A\"" w682 {
                      tunnel: w687 -> [w706 w710 w715 w719]
                      tunnel: TRUE -> [w707 w711 w714 w718]
                      tunnel: w675 -> [w708 w712 w716 w720]
                      tunnel: [w705 w709 w713 w717] -> w677
                      frame "R", Default {
                        n217 = Bundle By Name(cluster=w708, "Update R"=w707, "R"=w706) -> (w705:refnum<class "Supervisor.lvclass">)
                      }
                      frame "Q" {
                        n218 = Bundle By Name(cluster=w712, "Update Q"=w711, "Q"=w710) -> (w709:refnum<class "Supervisor.lvclass">)
                      }
                      frame "I" {
                        n219 = Bundle By Name(cluster=w716, "Update KI"=w714, "KI"=w715) -> (w713:refnum<class "Supervisor.lvclass">)
                      }
                      frame "A" {
                        n220 = Bundle By Name(cluster=w720, "KA"=w719, "Update KA"=w718) -> (w717:refnum<class "Supervisor.lvclass">)
                      }
                    }
                    n221 = String Length(string=w683) -> (length=w693:i32)
                    n222 = Greater?(x=w693, y=1) -> (0:w691:bool)
                  }
                }
                frame "PNO" {
                  # "TODO: Must be changed to work with GUI"
                  n223 = while {
                    shift-right: [w729] -> _
                    shift-left: w725 -> [w742]
                    shift-right: [w726] -> w723
                    shift-left: w724 -> [w726]
                    shift-right: [w727] -> w721
                    shift-left: w722 -> [w728]
                    stop <- w738 continue-if-true
                    n224 = Search/Split String(string=w742, search string/char (-)=",") -> (substring before match=w736:string, match + rest of string=w730:string)  [unwired: 1 in, 1 out]
                    n225 = Scan From String(format string="%1s:%1s", input string=w736, error in=w728) -> (remaining string=w735:string, error out=w727:errorcluster, output 1=w732:string, output 2=w733:string)  [unwired: 3 in, 1 out]
                    n226 = Replace Substring(2:1 ("length (len. of substring)"), 5:w730) -> (1:w729:string)  [unwired: 2 in, 1 out]
                    n227 = case shown="\"N\", Default" w732 {
                      tunnel: w735 -> [w745 w748]
                      tunnel: [w743 w746] -> w734
                      frame "N", Default {
                        n228 = call "String to Matrix (Norm).vi"("Martix Dimension"=6, "String"=w745) -> ("Output Matrix"=w743:T9)
                      }
                      frame "D" {
                        n229 = call "String to Matrix (Diag).vi"("Martix Dimension"=6, "String Input"=w748) -> ("Matrix Out"=w746:T9)
                      }
                    }
                    n230 = case shown="\"P\", Default" w733 {
                      tunnel: w734 -> [_ _ _ _]
                      frame "P", Default {
                      }
                      frame "D" {
                      }
                      frame "I" {
                      }
                      frame "A" {
                      }
                    }
                    n231 = String Length(string=w729) -> (length=w740:i32)
                    n232 = Greater?(x=w740, y=1) -> (0:w738:bool)
                  }
                }
              }
            }
            frame 20 {
              n233 = Scan From String(format string="%d", input string=w756, error in=w750) -> (error out=w749:errorcluster, output 1=w754:i32)  [unwired: 2 in, 2 out]
              n234 = Not Equal To 0?(x=w754) -> (x != 0?=w752:bool)
              n235 = Bundle By Name(cluster=w753, "MTi Active"=w752) -> (w751:refnum<class "Supervisor.lvclass">)
            }
            frame 21 {
              n236 = Scan From String(format string="%d", input string=w764, error in=w758) -> (error out=w757:errorcluster, output 1=w762:i32)  [unwired: 2 in, 2 out]
              n237 = Not Equal To 0?(x=w762) -> (x != 0?=w760:bool)
              n238 = Bundle By Name(cluster=w761, "MTi Gyro"=w760) -> (w759:refnum<class "Supervisor.lvclass">)
            }
            frame 22 {
              n239 = Scan From String(format string="%d", input string=w769, error in=w770) -> (error out=w765:errorcluster, output 1=w771:i32)  [unwired: 2 in, 2 out]
              n240 = Not Equal To 0?(x=w771) -> (x != 0?=w767:bool)
              n241 = Bundle By Name(cluster=w768, "Auto Parameter Reference Model Omega"=w767) -> (w766:refnum<class "Supervisor.lvclass">)
            }
            frame 23 {
              w775 = u16 2 ("Control Mode")
              n242 = Bundle By Name(cluster=w776, "Operation Type"=w775, "Control Mode"=w775) -> (w774:refnum<class "Supervisor.lvclass">)
            }
            frame 24 {
              n243 = Scan From String(format string="%d", input string=w782, error in=w781) -> (error out=w780:errorcluster, output 1=w783:i32)  [unwired: 2 in, 2 out]
              n244 = Not Equal To 0?(x=w783) -> (x != 0?=w778:bool)
              n245 = Bundle By Name(cluster=w779, "Use Chair Joystick"=w778) -> (w777:refnum<class "Supervisor.lvclass">)
            }
            frame 25 {
              n246 = Scan From String(format string="%d", input string=w790, error in=w786) -> (error out=w785:errorcluster, output 1=w788:i32)  [unwired: 2 in, 2 out]
              n247 = Not Equal To 0?(x=w788) -> (x != 0?=w787:bool)
              n248 = Bundle By Name(cluster=w792, "HPR"=w787) -> (w791:refnum<class "Supervisor.lvclass">)
            }
            frame 26 {
              n249 = Scan From String(format string="%d", input string=w795, error in=w794) -> (error out=w793:errorcluster, output 1=w799:i32)  [unwired: 2 in, 2 out]
              n250 = Not Equal To 0?(x=w799) -> (x != 0?=w800:bool)
              n251 = Bundle By Name(cluster=w797, "Sonar 1"=w800) -> (w796:refnum<class "Supervisor.lvclass">)
            }
            frame 27 {
              n252 = Scan From String(format string="%d", input string=w805, error in=w802) -> (error out=w801:errorcluster, output 1=w807:i32)  [unwired: 2 in, 2 out]
              n253 = Not Equal To 0?(x=w807) -> (x != 0?=w808:bool)
              n254 = Bundle By Name(cluster=w804, "Sonar 2"=w808) -> (w803:refnum<class "Supervisor.lvclass">)
            }
            frame 28 {
              n255 = Scan From String(format string="%d", input string=w809, error in=w811) -> (error out=w810:errorcluster, output 1=w815:i32)  [unwired: 2 in, 2 out]
              n256 = Not Equal To 0?(x=w815) -> (x != 0?=w814:bool)
              n257 = Bundle By Name(cluster=w813, "Doppler"=w814) -> (w812:refnum<class "Supervisor.lvclass">)
            }
            frame 29 {
              n258 = Scan From String(format string="%d", input string=w817, error in=w819) -> (error out=w818:errorcluster, output 1=w823:i32)  [unwired: 2 in, 2 out]
              n259 = Not Equal To 0?(x=w823) -> (x != 0?=w822:bool)
              n260 = Bundle By Name(cluster=w821, "Laser"=w822) -> (w820:refnum<class "Supervisor.lvclass">)
            }
            frame 30 {
              n261 = Scan From String(format string="%d", input string=w827, error in=w826) -> (error out=w825:errorcluster, output 1=w831:i32)  [unwired: 2 in, 2 out]
              n262 = Not Equal To 0?(x=w831) -> (x != 0?=w832:bool)
              n263 = Bundle By Name(cluster=w829, "KRAFT"=w832) -> (w828:refnum<class "Supervisor.lvclass">)
            }
            frame 31 {
              n264 = Scan From String(format string="%d", input string=w835, error in=w834) -> (error out=w833:errorcluster, output 1=w839:i32)  [unwired: 2 in, 2 out]
              n265 = Not Equal To 0?(x=w839) -> (x != 0?=w838:bool)
              n266 = Bundle By Name(cluster=w837, "Pan/Tilt"=w838) -> (w836:refnum<class "Supervisor.lvclass">)
            }
            frame 32 {
              n267 = Scan From String(format string="%d", input string=w843, error in=w844) -> (error out=w842:errorcluster, output 1=w847:i32)  [unwired: 2 in, 2 out]
              n268 = Not Equal To 0?(x=w847) -> (x != 0?=w846:bool)
              n269 = Bundle By Name(cluster=w845, "Transponder"=w846) -> (w841:refnum<class "Supervisor.lvclass">)
            }
            frame 33 {
              n270 = Scan From String(format string="%d", input string=w851, error in=w850) -> (error out=w849:errorcluster, output 1=w855:i32)  [unwired: 2 in, 2 out]
              n271 = Not Equal To 0?(x=w855) -> (x != 0?=w854:bool)
              n272 = Bundle By Name(cluster=w853, "Still Cam"=w854) -> (w852:refnum<class "Supervisor.lvclass">)
            }
            frame 34 {
              n273 = Scan From String(format string="%d", input string=w859, error in=w858) -> (error out=w857:errorcluster, output 1=w863:i32)  [unwired: 2 in, 2 out]
              n274 = Not Equal To 0?(x=w863) -> (x != 0?=w862:bool)
              n275 = Bundle By Name(cluster=w861, "HD Cam"=w862) -> (w860:refnum<class "Supervisor.lvclass">)
            }
            frame 35 {
              n276 = Scan From String(format string="%2s,%d", input string=w872, error in=w871) -> (error out=w870:errorcluster, output 1=w869:string, output 2=w868:i32)  [unwired: 3 in, 2 out]
              n277 = Not Equal To 0?(x=w868) -> (x != 0?=w866:bool)
              n278 = case shown="\"OU\"" w869 {
                tunnel: w867 -> [w876 w879 w882 w885 w888 w891 w894 w897 w900 w903]
                tunnel: w866 -> [w874 w877 w880 w883 w886 w889 w892 w895 w899 w902]
                tunnel: [w875 w878 w881 w884 w887 w890 w893 w896 w898 w901] -> w865
                frame "IN", Default {
                  n279 = Bundle By Name(cluster=w876, "In"=w874) -> (w875:refnum<class "Supervisor.lvclass">)
                }
                frame "PP" {
                  n280 = Bundle By Name(cluster=w879, "Pressure +"=w877) -> (w878:refnum<class "Supervisor.lvclass">)
                }
                frame "PM" {
                  n281 = Bundle By Name(cluster=w882, "Pressure -"=w880) -> (w881:refnum<class "Supervisor.lvclass">)
                }
                frame "VP" {
                  n282 = Bundle By Name(cluster=w885, "Vacuum +"=w883) -> (w884:refnum<class "Supervisor.lvclass">)
                }
                frame "VM" {
                  n283 = Bundle By Name(cluster=w888, "Vacuum -"=w886) -> (w887:refnum<class "Supervisor.lvclass">)
                }
                frame "OU" {
                  n284 = Bundle By Name(cluster=w891, "Out"=w889) -> (w890:refnum<class "Supervisor.lvclass">)
                }
                frame "TO" {
                  n285 = Bundle By Name(cluster=w894, "To"=w892) -> (w893:refnum<class "Supervisor.lvclass">)
                }
                frame "FR" {
                  n286 = Bundle By Name(cluster=w897, "From"=w895) -> (w896:refnum<class "Supervisor.lvclass">)
                }
                frame "CC" {
                  n287 = Bundle By Name(cluster=w900, "Rotate CCW"=w899) -> (w898:refnum<class "Supervisor.lvclass">)
                }
                frame "CW" {
                  n288 = Bundle By Name(cluster=w903, "Rotate CW"=w902) -> (w901:refnum<class "Supervisor.lvclass">)
                }
              }
            }
            frame 36 {
              n289 = Scan From String(format string="%d", input string=w911, error in=w905) -> (error out=w904:errorcluster, output 1=w909:i32)  [unwired: 2 in, 2 out]
              n290 = Not Equal To 0?(x=w909) -> (x != 0?=w907:bool)
              n291 = Bundle By Name(cluster=w908, "Only New HiPAP"=w907) -> (w906:refnum<class "Supervisor.lvclass">)
            }
            frame 37 {
              n292 = Scan From String(format string="%d", input string=w919, error in=w917) -> (error out=w915:errorcluster, output 1=w916:i32)  [unwired: 2 in, 2 out]
              n293 = Not Equal To 0?(x=w916) -> (x != 0?=w913:bool)
              n294 = Bundle By Name(cluster=w914, "Reset SP"=w913) -> (w912:refnum<class "Supervisor.lvclass">)
            }
            frame 38 {
              w930 = ""
              n295 = Unbundle By Name(w923) -> ("Controllers"=w932:string[], "Observers"=w931:string[])
              n296 = for {
                tunnel: w931 -> [w935] mode=indexing
                shift-right: [w934] -> w929
                shift-left: w930 -> [w933]
                n297 = call "Build Text3"("Beginning Text"=w933, "Input"=w935) -> ("Result"=w934:string)  [unwired: 12 in, 1 out]
              }
              n298 = for {
                tunnel: w932 -> [w938] mode=indexing
                shift-right: [w937] -> w928
                shift-left: w930 -> [w936]
                n299 = call "Build Text"("Beginning Text"=w936, "Input"=w938) -> ("Result"=w937:string)  [unwired: 12 in, 1 out]
              }
              n300 = call "Build Text4"("Controllers"=w928, "Observers"=w929) -> ("Result"=w925:string)  [unwired: 12 in, 1 out]
              n301 = String Length(string=w925) -> (length=w927:i32)
              n302 = Type Cast(type=w925, x=w927) -> (*(type *) &x=w926:string)
              n303 = Concatenate Strings(w926, w925) -> (w924:string)
              n304 = TCP Write(connection ID=w920, data in=w924, error in (no error)=w922) -> (error out=w921:errorcluster)  [unwired: 1 in, 2 out]
            }
            frame 39 {
              n305 = Scan From String(format string="%d,", input string=w943) -> (remaining string=w942:string, output 1=w944:i32)  [unwired: 3 in, 2 out]
              n306 = Not Equal To 0?(x=w944) -> (x != 0?=w941:bool)
              n307 = case shown="False" w941 {
                selector: w941 -> [w948 w954]
                tunnel: w947 -> [w950 w961]
                tunnel: w946 -> [w949 w959]
                tunnel: w942 -> [_ w955]
                tunnel: [w951 w953] -> w940
                tunnel: [w950 w952] -> w939
                frame False {
                  n308 = Bundle By Name(cluster=w949, "Use Altitude Guidance"=w948, "Reset Reference Model"=w948) -> (w951:refnum<class "Supervisor.lvclass">)
                }
                frame True {
                  n309 = Scan From String(format string="%d,%d,%f", input string=w955, error in=w961) -> (error out=w952:errorcluster, output 1=w962:i32, output 2=w960:i32, output 3=w956:dbl)  [unwired: 4 in, 2 out]
                  n310 = Not Equal To 0?(x=w962) -> (x != 0?=w958:bool)
                  n311 = Not Equal To 0?(x=w960) -> (x != 0?=w957:bool)
                  n312 = Bundle By Name(cluster=w959, "Use Integrator"=w958, "Use FeedForward"=w957, "Reset Reference Model"=w954, "Desired Altitude"=w956, "Use Altitude Guidance"=w954) -> (w953:refnum<class "Supervisor.lvclass">)
                }
              }
            }
            frame 40 {
              n313 = Scan From String(format string="%d", input string=w967, error in=w969) -> (error out=w965:errorcluster, output 1=w964:i32)  [unwired: 2 in, 2 out]
              n314 = Bundle By Name(cluster=w968, "Joystick Response"=w964) -> (w966:refnum<class "Supervisor.lvclass">)
            }
            frame 41 {
              n315 = Scan From String(format string="%d", input string=w976, error in=w975) -> (error out=w972:errorcluster)  [unwired: 3 in, 2 out]
              n316 = Bundle By Name(cluster=w974, "Break"=TRUE ("CJ Cluster.Break")) -> (w973:refnum<class "Supervisor.lvclass">)
            }
            frame 42 {
              n317 = Scan From String(format string="%f,%f", input string=w997, error in=w996) -> (error out=w984:errorcluster, output 1=w980:dbl, output 2=w979:dbl)  [unwired: 3 in, 2 out]
              n318 = call-dynamic "Read CJ Cluster.vi"("error in (no error)"=w984, "Supervisor in"=w985) -> ("error out"=w983:errorcluster, "CJ Cluster"=w989:T1, "Supervisor out"=w986:refnum<class "Supervisor.lvclass">)  [unwired: 7 in]
              n319 = expression code="(x/180.0)*pi" ("degrees to radians")(w979) -> (w978:dbl)
              n320 = Build Array(0.1 ("element"), 0.1 ("element"), w980) -> (w991:dbl[])
              n321 = Build Array(0.2 ("element"), 0.2 ("element"), w978) -> (w990:dbl[])
              n322 = Bundle(cluster=w989, "javp"=w991, "javr"=w990, "Break"=FALSE ("Guidance Cluster.Update Reference.Mode Change")) -> (w988:T1)  [unwired: 2 in]
              n323 = call-dynamic "Write CJ Cluster.vi"("error in (no error)"=w983, "CJ Cluster"=w988, "Supervisor in"=w986) -> ("error out"=w981:errorcluster, "Supervisor out"=w982:refnum<class "Supervisor.lvclass">)  [unwired: 7 in]
            }
            frame 43 {
              n324 = Scan From String(format string="%d", input string=w1008, error in=w1009) -> (error out=w1002:errorcluster, output 1=w1004:i32)  [unwired: 2 in, 2 out]
              n325 = call-dynamic "Read Tracking Cluster.vi"("error in (no error)"=w1002, "Supervisor in"=w1007) -> ("error out"=w1001:errorcluster, "Tracking Cluster"=w1006:T10, "Supervisor out"=w1003:refnum<class "Supervisor.lvclass">)  [unwired: 7 in]
              n326 = Bundle By Name(cluster=w1006, "Heading Mode"=w1004) -> (w1005:T10)
              n327 = call-dynamic "Write Tracking Cluster.vi"("error in (no error)"=w1001, "Tracking Cluster"=w1005, "Supervisor in"=w1003) -> ("error out"=w999:errorcluster, "Supervisor out"=w1000:refnum<class "Supervisor.lvclass">)  [unwired: 7 in]
            }
            frame 44 {
              n328 = Scan From String(format string="%f", input string=w1016, error in=w1017) -> (error out=w1019:errorcluster, output 1=w1012:dbl)  [unwired: 2 in, 2 out]
              n329 = call-dynamic "Read Tracking Cluster.vi"("error in (no error)"=w1019, "Supervisor in"=w1015) -> ("error out"=w1018:errorcluster, "Tracking Cluster"=w1022:T10, "Supervisor out"=w1020:refnum<class "Supervisor.lvclass">)  [unwired: 7 in]
              n330 = expression code="(x/180.0)*pi" "degrees to radians"(w1012) -> (w1011:dbl)
              n331 = Bundle By Name(cluster=w1022, "Tracking Options.(2) Fixed Heading"=w1011) -> (w1021:T10)
              n332 = call-dynamic "Write Tracking Cluster.vi"("error in (no error)"=w1018, "Tracking Cluster"=w1021, "Supervisor in"=w1020) -> ("error out"=w1014:errorcluster, "Supervisor out"=w1013:refnum<class "Supervisor.lvclass">)  [unwired: 7 in]
            }
            frame 45 {
              n333 = Scan From String(format string="%f,%f,%f", input string=w1033, error in=w1032) -> (error out=w1026:errorcluster, output 1=w1030:dbl, output 2=w1029:dbl, output 3=w1028:dbl)  [unwired: 4 in, 2 out]
              n334 = Build Array(w1030, w1029, w1028) -> (w1027:dbl[])
              n335 = call-dynamic "Write r_offset.vi"("error in (no error)"=w1026, "r_offset"=w1027, "Supervisor in"=w1031) -> ("error out"=w1025:errorcluster, "Supervisor out"=w1024:refnum<class "Supervisor.lvclass">)  [unwired: 7 in]
            }
            frame 47 {
              n336 = Scan From String(format string="%d", input string=w1039, error in=w1038) -> (error out=w1036:errorcluster, output 1=w1041:i32)  [unwired: 2 in, 2 out]
              n337 = Not Equal To 0?(x=w1041) -> (x != 0?=w1042:bool)
              n338 = Bundle By Name(cluster=w1037, "DVL Direct"=w1042) -> (w1035:refnum<class "Supervisor.lvclass">)
            }
            frame 48 {
              n339 = Scan From String(format string="%d", input string=w1048, error in=w1047) -> (error out=w1046:errorcluster, output 1=w1044:i32)  [unwired: 2 in, 2 out]
              n340 = Bundle By Name(cluster=w1043, "Pressure Mode"=w1044) -> (w1045:refnum<class "Supervisor.lvclass">)
            }
            frame 49 {
              n341 = Scan From String(format string="%d", input string=w1056, error in=w1052) -> (error out=w1051:errorcluster, output 1=w1055:i32)  [unwired: 2 in, 2 out]
              n342 = call-dynamic "Write Observer type.vi"("error in (no error)"=w1051, "Observer type"=w1055, "Supervisor in"=w1054) -> ("error out"=w1050:errorcluster, "Supervisor out"=w1053:refnum<class "Supervisor.lvclass">)  [unwired: 7 in]
            }
            frame 50 {
              # "This code takes the gains of the KF from the supervisor class and writes down the values of the matrices in\na string with the following standard:\nrXXcYY;ZZ,nnn,nnn,nnn,nnn ...................;\nrXX'cYY';ZZ',nnn',nnn',nnn',nnn' ...................;\nthe entries are scanned through rows. n1,n2,n3;\n                                                                   n4,n5,n6."
              n343 = call-dynamic "Read Kalman Filter Observer Tuning.vi"("Supervisor in"=w1086) -> ("Kalman Filter Observer Tuning"=w1085:T11)  [unwired: 8 in, 2 out]
              n344 = Unbundle(w1085) -> ("R"=w1080:T9, "Q"=w1060:T9)  [unwired: 3 out]
              n345 = Matrix Size(0:w1080) -> (1:w1079:i32, 2:w1078:i32)
              n346 = Matrix Size(0:w1060) -> (1:w1077:i32, 2:w1076:i32)
              n347 = Number To Decimal String(number=w1079) -> (decimal integer string=w1075:string)  [unwired: 1 in]
              n348 = Number To Decimal String(number=w1078) -> (decimal integer string=w1074:string)  [unwired: 1 in]
              n349 = Number To Decimal String(number=w1077) -> (decimal integer string=w1067:string)  [unwired: 1 in]
              n350 = Number To Decimal String(number=w1076) -> (decimal integer string=w1066:string)  [unwired: 1 in]
              n351 = Concatenate Strings("r" ("String"), w1075, "c" ("String"), w1074) -> (w1061:string)
              n352 = Concatenate Strings(w1061, ";" ("String"), "R" ("String")) -> (w1070:string)
              n353 = call "MatrixToString.vi"("Header (default: no header)"=w1070, "Matrix in"=w1080) -> ("String out"=w1082:string)  [unwired: 9 in]
              n354 = Concatenate Strings("r" ("String"), w1067, "c" ("String"), w1066) -> (w1064:string)
              n355 = Concatenate Strings(w1064, ";" ("String"), "Q") -> (w1059:string)
              n356 = call "MatrixToString.vi"("Header (default: no header)"=w1059, "Matrix in"=w1060) -> ("String out"=w1058:string)  [unwired: 9 in]
              n357 = call "Build Text6"("Input"=w1058) -> ("Result"=w1084:string)  [unwired: 13 in, 1 out]
              n358 = call "Build Text5"("Input"=w1082) -> ("Result"=w1083:string)  [unwired: 13 in, 1 out]
              n359 = call "Build Text8"("R"=w1083, "Q"=w1084) -> ("Result"=w1081:string)  [unwired: 12 in, 1 out]
              n360 = String Length(string=w1081) -> (length=w1092:i32)
              n361 = Type Cast(type=w1081, x=w1092) -> (*(type *) &x=w1091:string)
              n362 = Concatenate Strings(w1091, w1081) -> (w1090:string)
              n363 = TCP Write(connection ID=w1089, data in=w1090, error in (no error)=w1088) -> (error out=w1087:errorcluster)  [unwired: 1 in, 2 out]
            }
            frame 51 {
              # "This code takes the gains of the KF from the supervisor class and writes down the values of the matrices in\na string with the following standard:\nrXXcYY;ZZ,nnn,nnn,nnn,nnn ...................;\nrXX'cYY';ZZ',nnn',nnn',nnn',nnn' ...................;\nthe entries are scanned through rows. n1,n2,n3;\n                                                                   n4,n5,n6."
              n364 = call-dynamic "Read Non Linear PID Tuning.vi"("Supervisor in"=w1122) -> ("Non Linear PID Tuning"=w1121:T12)  [unwired: 8 in, 2 out]
              n365 = Unbundle(w1121) -> ("KP"=w1120:T9, "KD"=w1119:T9, "KI"=w1098:T9, "KA"=w1097:T9)  [unwired: 5 out]
              n366 = Matrix Size(0:w1120) -> (1:w1143:i32, 2:w1142:i32)
              n367 = Matrix Size(0:w1119) -> (1:w1141:i32, 2:w1140:i32)
              n368 = Matrix Size(0:w1098) -> (1:w1107:i32, 2:w1108:i32)
              n369 = Matrix Size(0:w1097) -> (1:w1109:i32, 2:w1110:i32)
              n370 = Number To Decimal String(number=w1143) -> (decimal integer string=w1139:string)  [unwired: 1 in]
              n371 = Number To Decimal String(number=w1107) -> (decimal integer string=w1111:string)  [unwired: 1 in]
              n372 = Number To Decimal String(number=w1142) -> (decimal integer string=w1138:string)  [unwired: 1 in]
              n373 = Number To Decimal String(number=w1108) -> (decimal integer string=w1112:string)  [unwired: 1 in]
              n374 = Number To Decimal String(number=w1141) -> (decimal integer string=w1131:string)  [unwired: 1 in]
              n375 = Number To Decimal String(number=w1109) -> (decimal integer string=w1117:string)  [unwired: 1 in]
              n376 = Number To Decimal String(number=w1140) -> (decimal integer string=w1130:string)  [unwired: 1 in]
              n377 = Number To Decimal String(number=w1110) -> (decimal integer string=w1118:string)  [unwired: 1 in]
              n378 = Concatenate Strings("r" ("String"), w1139, "c" ("String"), w1138) -> (w1125:string)
              n379 = Concatenate Strings(w1125, ";" ("String"), "P" ("String")) -> (w1134:string)
              n380 = call "MatrixToString.vi"("Header (default: no header)"=w1134, "Matrix in"=w1120) -> ("String out"=w1145:string)  [unwired: 9 in]
              n381 = Concatenate Strings("r" ("String"), w1111, "c" ("String"), w1112) -> (w1102:string)
              n382 = Concatenate Strings(w1102, ";" ("String"), "I") -> (w1096:string)
              n383 = call "MatrixToString.vi"("Header (default: no header)"=w1096, "Matrix in"=w1098) -> ("String out"=w1094:string)  [unwired: 9 in]
              n384 = Concatenate Strings("r" ("String"), w1131, "c" ("String"), w1130) -> (w1128:string)
              n385 = Concatenate Strings(w1128, ";" ("String"), "D") -> (w1124:string)
              n386 = call "MatrixToString.vi"("Header (default: no header)"=w1124, "Matrix in"=w1119) -> ("String out"=w1123:string)  [unwired: 9 in]
              n387 = Concatenate Strings("r" ("String"), w1117, "c" ("String"), w1118) -> (w1101:string)
              n388 = Concatenate Strings(w1101, ";" ("String"), "A") -> (w1095:string)
              n389 = call "MatrixToString.vi"("Header (default: no header)"=w1095, "Matrix in"=w1097) -> ("String out"=w1093:string)  [unwired: 9 in]
              n390 = call "Build Text12"("Input"=w1093) -> ("Result"=w1099:string)  [unwired: 13 in, 1 out]
              n391 = call "Build Text10"("Input"=w1123) -> ("Result"=w1147:string)  [unwired: 13 in, 1 out]
              n392 = call "Build Text11"("Input"=w1094) -> ("Result"=w1100:string)  [unwired: 13 in, 1 out]
              n393 = call "Build Text9"("Input"=w1145) -> ("Result"=w1146:string)  [unwired: 13 in, 1 out]
              n394 = call "Build Text7"("KA"=w1099, "KP"=w1146, "KD"=w1147, "KI"=w1100) -> ("Result"=w1144:string)  [unwired: 10 in, 1 out]
              n395 = String Length(string=w1144) -> (length=w1153:i32)
              n396 = Type Cast(type=w1144, x=w1153) -> (*(type *) &x=w1152:string)
              n397 = Concatenate Strings(w1152, w1144) -> (w1151:string)
              n398 = TCP Write(connection ID=w1150, data in=w1151, error in (no error)=w1149) -> (error out=w1148:errorcluster)  [unwired: 1 in, 2 out]
            }
            frame 52 {
              n399 = Scan From String(format string="%d", input string=w1157, error in=w1156) -> (error out=w1155:errorcluster, output 1=w1158:i32)  [unwired: 2 in, 2 out]
              n400 = Not Equal To 0?(x=w1158) -> (x != 0?=w1154:bool)
              n401 = call-dynamic "Write Reset Pressure.vi"("error in (no error)"=w1155, "Reset Pressure"=w1154, "Supervisor in"=w1161) -> ("error out"=w1162:errorcluster, "Supervisor out"=w1160:refnum<class "Supervisor.lvclass">)  [unwired: 7 in]
            }
            frame 53 {
              n402 = Scan From String(format string="%f", input string=w1164, error in=w1168) -> (error out=w1167:errorcluster, output 1=w1165:dbl)  [unwired: 2 in, 2 out]
              n403 = call-dynamic "Write Atmospheric Pressure (kPa).vi"("error in (no error)"=w1167, "Atmospheric Pressure (deciBar)"=w1165, "Supervisor in"=w1169) -> ("error out"=w1166:errorcluster, "Supervisor out"=w1163:refnum<class "Supervisor.lvclass">)  [unwired: 7 in]
            }
            frame 54 {
              n404 = Scan From String(format string="%d", input string=w1176, error in=w1177) -> (error out=w1172:errorcluster, output 1=w1178:i32)  [unwired: 2 in, 2 out]
              n405 = Not Equal To 0?(x=w1178) -> (x != 0?=w1175:bool)
              n406 = call-dynamic "Write Manual Reset.vi"("error in (no error)"=w1172, "Manual Reset"=w1175, "Supervisor in"=w1174) -> ("error out"=w1171:errorcluster, "Supervisor out"=w1173:refnum<class "Supervisor.lvclass">)  [unwired: 7 in]
            }
            frame 55 {
              n407 = Scan From String(format string="%d", input string=w1186, error in=w1185) -> (error out=w1181:errorcluster, output 1=w1188:i32)  [unwired: 2 in, 2 out]
              n408 = Not Equal To 0?(x=w1188) -> (x != 0?=w1182:bool)
              n409 = call-dynamic "Write Start New LogFile.vi"("error in (no error)"=w1181, "Start New LogFile"=w1182, "Supervisor in"=w1183) -> ("error out"=w1180:errorcluster, "Supervisor out"=w1184:refnum<class "Supervisor.lvclass">)  [unwired: 7 in]
            }
            frame 56 {
              n410 = Scan From String(format string="%d", input string=w1191, error in=w1192) -> (error out=w1193:errorcluster, output 1=w1195:i32)  [unwired: 2 in, 2 out]
              n411 = Not Equal To 0?(x=w1195) -> (x != 0?=w1194:bool)
              n412 = Bundle By Name(cluster=w1190, "UHI Cam"=w1194) -> (w1189:refnum<class "Supervisor.lvclass">)
            }
            frame 57 {
              n413 = Scan From String(format string="%f", input string=w1202, error in=w1203) -> (error out=w1200:errorcluster, output 1=w1201:dbl)  [unwired: 2 in, 2 out]
              n414 = call-dynamic "Write Latitude for UNI-Depth calculation.vi"("error in (no error)"=w1200, "Latitude for UNI-Depth calculation"=w1201, "Supervisor in"=w1199) -> ("error out"=w1198:errorcluster, "Supervisor out"=w1197:refnum<class "Supervisor.lvclass">)  [unwired: 7 in]
            }
          }
        }
      }
    }
    frame Error {
      n415 = Unbundle By Name(w1206) -> ("code"=w1209:i32)
      n416 = case shown="66" w1209 {
        tunnel: w1206 -> [w1212 w1214]
        tunnel: w1208 -> [w1211 w1213]
        tunnel: [w1211 w1213] -> w1207
        tunnel: [w1212 w1214] -> w1205
        frame 0, Default {
        }
        frame 66 {
        }
      }
    }
  }
  "TCP Network Connection Refnum Out" <- w14
  "Supervisor Out" <- w13
  "Error Out" <- w11
